vi "Text control 2 v6.1.vi"() -> ()   [LabVIEW 2016]
panel:
  in  "Tab Control":enum32{"Main", "Other parameters"}(tab)
  out "Line running":i32
  out "Total lines":i32
  out "Path":path=path "C:/users/rlp38/09Apr2009LTtesting/test2.txt"
  out "I vs Vg":cluster{"Y data in":dbl[], "X data in":dbl[]}[](graph)
  out "Is max":dbl format="%.2e"
  out "Id max":dbl format="%.2e"
  out "Ig max":dbl format="%.2e"
  out "Imax vs time":cluster{"Y data in":dbl[], "X data in":dbl[]}[](graph)
  out "Imin vs time":cluster{"Y data in":dbl[], "X data in":dbl[]}[](graph)
  out "I vs Vd":cluster{"Y data in":dbl[], "X data in":dbl[]}[](graph)
  in  "Script":string="#pulsedstressV d 0.03 20 0 0.5 0.0827 5\n#\n#itime m\n#gaterangemode a\n#drainrangemode a\n#pulsed on 0.05 0 0.02\n#transfer d -10 40 1 5 40 35\n#transfer d -10 40 1 5 40 35\n#transfer d -10 40 1 5 40 35\n#output d 0 40 20 0 40 1\n#\n#\n#sample 1 0.008 221 6 0.003\n#samplei 400e-6 200 6 0.002 0.1\n#vsu2pulse -10 4\n#\n#stressV 0.016 0.03 2e-4 0.1e-3 11\n#stressI 220e-7 0.08 15\n#transfer s -1 1 0.5 -0.005 0.005 0.005\n#output s 0 0 0 -0.008 0.008 0.002"
  out "Command running:":string
  out "Serial port data":string
  out "Elapsed Time":dbl caption="Elapsed Time (s)"
  in  "Time Units":u16(ring)=1 items=["Seconds", "Minutes", "Hours"]
  in  "Time Offset":dbl caption="Set Start Time (s)"
  in  "Reset":bool
  in  "Auto Reset":bool
  in  "integration time":u32(slide) max=2 step=1 scale=0.0..2.0
  out "Is on":dbl format="%.2e"
  out "Id on":dbl format="%.2e"
  out "Ig on":dbl format="%.2e"
  out "Ion vs time":cluster{"Y data in":dbl[], "X data in":dbl[]}[](graph)
  out "Ioff vs time":cluster{"Y data in":dbl[], "X data in":dbl[]}[](graph)
  out "Ig min":dbl format="%.2e"
  out "Id min":dbl format="%.2e"
  out "Is min":dbl format="%.2e"
  out "Is off":dbl format="%.2e"
  out "Id off":dbl format="%.2e"
  out "Ig off":dbl format="%.2e"
  in  "Integration time (long)":dbl=0.32 min=0.04 max=2.0 step=0.02 format="%.2f"
  in  "Integration time (short)":dbl=0.0019 min=8e-05 max=0.0019 step=8e-05 format="%^.0e"
  in  "Drain: Compliance":dbl=0.001 format="%.8f"
  in  "Gate: Compliance":dbl=0.001 format="%.8f"
  in  "Interrupt run":bool
  in  "Standby":T1
  in  "Full Reset":bool
  in  "SMU4":cluster{"on/off":bool, "Voltage":dbl} {"Voltage" min=-100.0 max=100.0 format="%.2f"}
  in  "Gate Range\nmode":u16(ring) items=["Auto", "Limited", "Fixed"]
  in  "Gate Range":u8(slide)=6 max=11 scale=0.0..11.0
  in  "Source/Drain\nRange mode":u16(ring) items=["Auto", "Limited", "Fixed"]
  in  "Source/Drain Range":u8(slide)=6 max=11 scale=0.0..11.0
  in  "Panel Controls":T2={"Emergency Stop"=refnum, "TransGraph Max"=1e-05, "Text/Graph (text=false)"=TRUE} {"TransGraph Max" format="%.2e"}
  in  "Panel Controls 2":T3={"Emergency Stop"=refnum, "TransGraph Max"=1e-05, "Text/Graph (text=false)"=TRUE, "TransGraph Min"=1e-11} {"TransGraph Min" format="%.2e"; "TransGraph Max" format="%.2e"}
  out "error out":errorcluster
  in  "Delay before read (ms)":u32=1000
  in  "byte count":u32=64
  in  "Serial End Mode for Reads":u16(ring)=2 items=["None", "LastBit", "TermChar"]
  in  "Timeout (ms)":u32=10000
  in  "Enable Termination\nChar (T)":bool=TRUE
  in  "Termination char\n(0xA = '\\n' = LF)\n(0xD = '\\r' = CR)":u8=13 format="%.0x"
  in  "flow control":u16(ring) items=["None"=0, "XON/XOFF"=1, "RTS/CTS"=2, "DTR/DSR"=4]
  in  "stop bits":u16(ring)=10 items=["1.0"=10, "1.5"=15, "2.0"=20]
  in  "parity":u16(ring) items=["None", "Odd", "Even", "Mark", "Space"]
  in  "data bits":u16=8 min=5 max=8 step=1
  in  "VISA resource name":refnum<visa-resource-name>="COM6"
  in  "baud rate":u32=9600
  out "Timings Indicator":T4
  in  "Timings (overwritten by the Front Panel)":T5={"integration time"=0, "Short/Long integration time"=0.00064, "hold time (sec)"=0.0, "delay time (sec)"=0.0, "Step Time (0 disables)"=0.0, "sweep method"=0, "Pulse period"=0.005, "Base voltage"=0.0, "Pulse width"=0.0005} {"Pulse width" min=0.0005 max=0.1 step=0.0001 format="%.4f"; "Base voltage" format="%^.4e"; "Pulse period" min=0.005 max=1.0 step=0.0001 format="%.4f"; "sweep method" items=["Continuous", "Pulsed"]; "Step Time (0 disables)" format="%.2f"; "delay time (sec)" format="%.4f"; "hold time (sec)" format="%.4f"; "Short/Long integration time" format="%^.0e"; "integration time" scale=0.0..2.0}
  in  "Gate":T6={"Gate Start"=0.0, "Gate Stop"=2.0, "Gate Step (linear only)"=1.0, "Gate Compliance"=0.0001, "Gate PComp"=0.0, "Range mode"=0, "Range"=6} {"Range" max=11 scale=0.0..11.0; "Range mode" items=["Auto", "Limited", "Fixed"]; "Gate PComp" format="%^.2e"; "Gate Compliance" format="%^.2e"; "Gate Step (linear only)" format="%^.4e"; "Gate Stop" format="%^.4e"; "Gate Start" format="%^.4e"}
  in  "Drain 2":T7={"Drain Start"=0.0, "Drain Stop"=2.0, "Drain Compliance"=0.0001, "Drain Step"=1.0, "Drain PComp"=0.0, "Range mode"=0, "Range"=6} {"Range" max=11 scale=0.0..11.0; "Range mode" items=["Auto", "Limited", "Fixed"]; "Drain PComp" format="%^.2e"; "Drain Step" format="%^.4e"; "Drain Compliance" format="%^.2e"; "Drain Stop" format="%^.4e"; "Drain Start" format="%^.4e"}
  # "Time"
  # "Syntax:\nitime [s|m|l] time(sec): [s|m|l] determines the integration time setting (small|medium|long) and time sets the value.\nNOTE: The value of the integration time has to be within the range allowed by its category (s|m|l), otherwise, the closest value will be used. (e.g. if the category is set to short but the time value is very long, the actual value used will be the maximum short integration time.\nIntegration times:\n    Short: Default: 640 us. Range: 8E-5 - 1.92E-3 seconds.\n    Medium: Fixed at 1 NPL cycle (0.02 seconds).\n    Long: Default: 16 NPL cycles (0.32 seconds). Range: 2-100 NPL cycles (0.04 seconds - 2 seconds).\ngaterangemode [a|l|f]\ndrainrangemode [a|l|f]\npulsed [on|off] PulsePeriod(sec) PulseBaseVoltage PulseONWidth(sec)\nstandby [on l off]\nwait NumMilliseconds\nwait-min NumMinutes\n# texthere = comment\ntransfer [s|d] VgStart VgStop VgStep VdStart VdStop VdStep\noutput [s|d] VgStart VgStop VgStep VdStart VdStop VdStep\nsample Vg Vd NumSamples Time(s) SampleInterval(s)\nsamplei Idg NumSamples Time(s) SampleInterval(s) VDGcompliance\n100 samples is approximately 13 seconds with medium integration\n# if in doubt use SampleInterval(s) = 0.004\nstressV VG VD IGcompliance IDcompliance Duration(sec)\nstressI IDG VDGcompliance Duration(sec)\nvsu2pulse Bias Duration(s)\npulsedstressV [s|d] VEstop VgON VgOFF Period(s) PulseONwidth(s) Vd\nsample-fpp Vg Vd NumSamples Time\nresample-fpp Vg Vd\ntransfer-fpp [s|d] VgStart VgStop VgStep VdStart VdStop VdStep\noutput-fpp [s|d] VgStart VgStop VgStep VdStart VdStop VdStep\nserial SerialPortCommand"
  # "1\n2\n3\n4\n5\n6\n7\n8\n9\n10\n11\n12\n13\n14\n15\n16\n17\n18\n19\n20"
  # "Serial port settings"
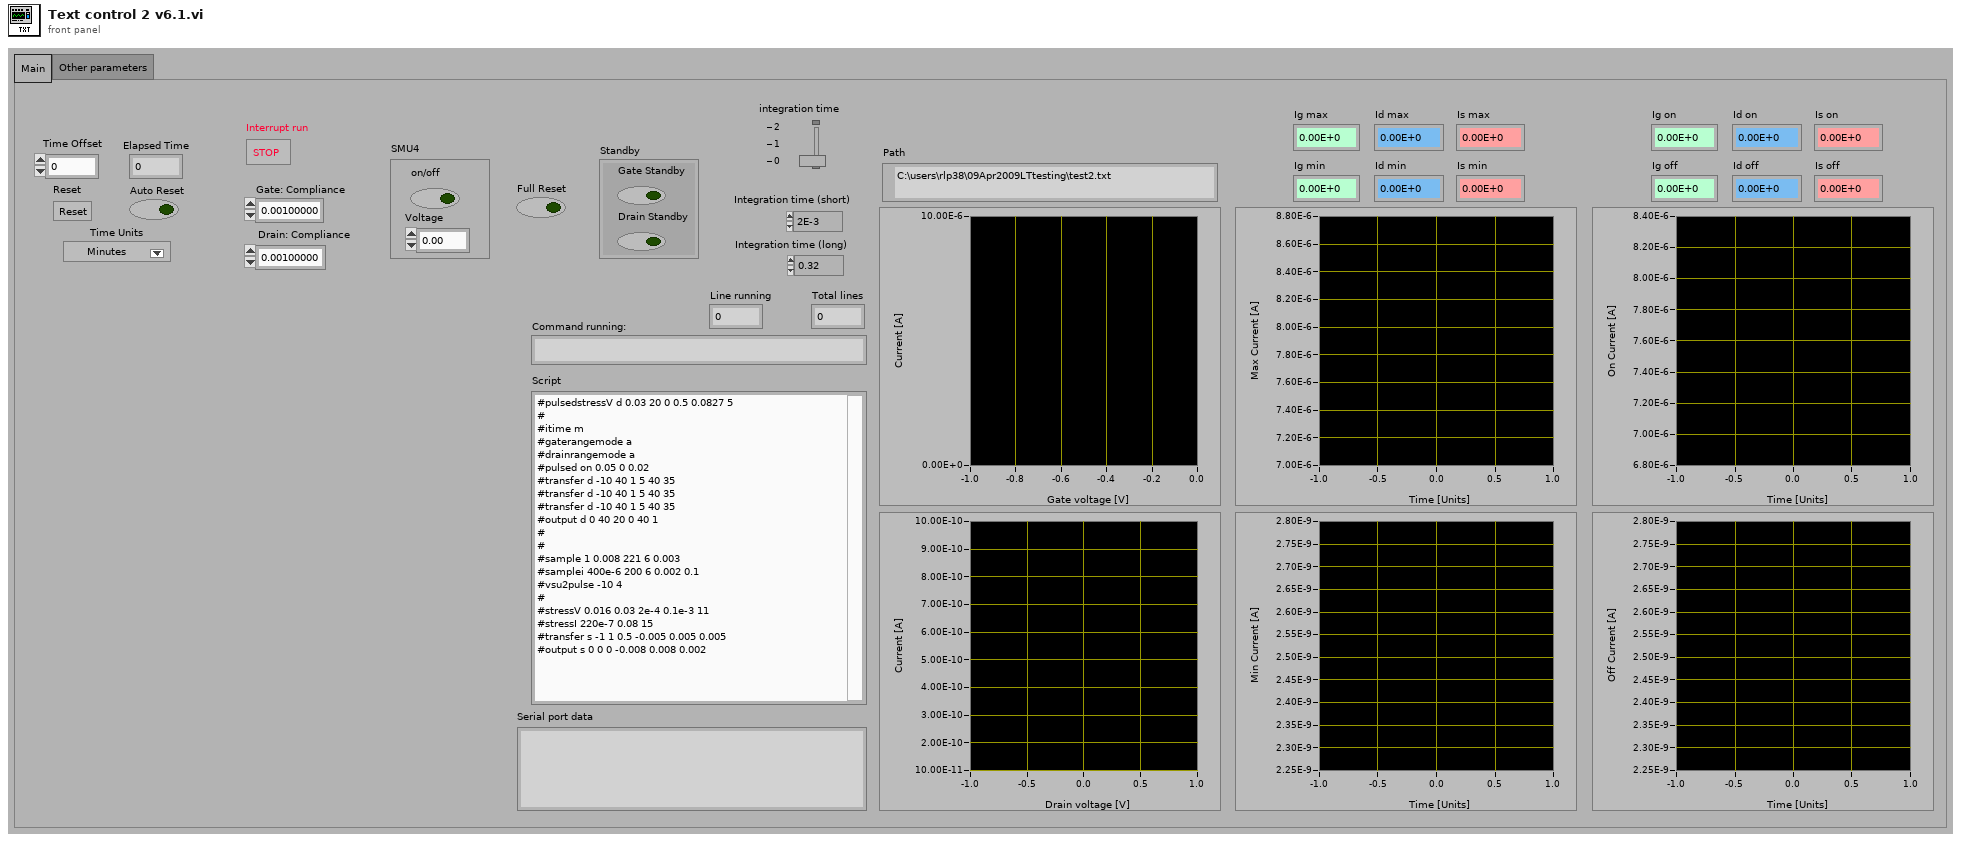
[diagram p1: front panel]
types:
  T1 = cluster{"Gate Standby":bool, "Drain Standby":bool}
  T2 = cluster{"Emergency Stop":refnum<vi>, "TransGraph Max":dbl, "Text/Graph (text=false)":bool}
  T3 = cluster{"Emergency Stop":refnum<vi>, "TransGraph Max":dbl, "Text/Graph (text=false)":bool, "TransGraph Min":dbl}
  T4 = cluster{"integration time (0:s, 1:m, 2:l)":u32, "Short/Long integration time":dbl, "hold time (sec)":dbl, "delay time (sec)":dbl, "Step Time (0 disables)":dbl, "sweep method":u16, "Pulse period":dbl, "Base voltage":dbl, "Pulse width":dbl}
  T5 = cluster{"integration time":u32, "Short/Long integration time":dbl, "hold time (sec)":dbl, "delay time (sec)":dbl, "Step Time (0 disables)":dbl, "sweep method":u16, "Pulse period":dbl, "Base voltage":dbl, "Pulse width":dbl}
  T6 = cluster{"Gate Start":dbl, "Gate Stop":dbl, "Gate Step (linear only)":dbl, "Gate Compliance":dbl, "Gate PComp":dbl, "Range mode":u16, "Range":u8}
  T7 = cluster{"Drain Start":dbl, "Drain Stop":dbl, "Drain Compliance":dbl, "Drain Step":dbl, "Drain PComp":dbl, "Range mode":u16, "Range":u8}
  T8 = enum16{"open", "replace", "create", "open or create", "replace or create", "replace or create with confirmation"}
  T9 = cluster{"V2 Start":dbl, "V2 Step":dbl, "Number of points":i32}
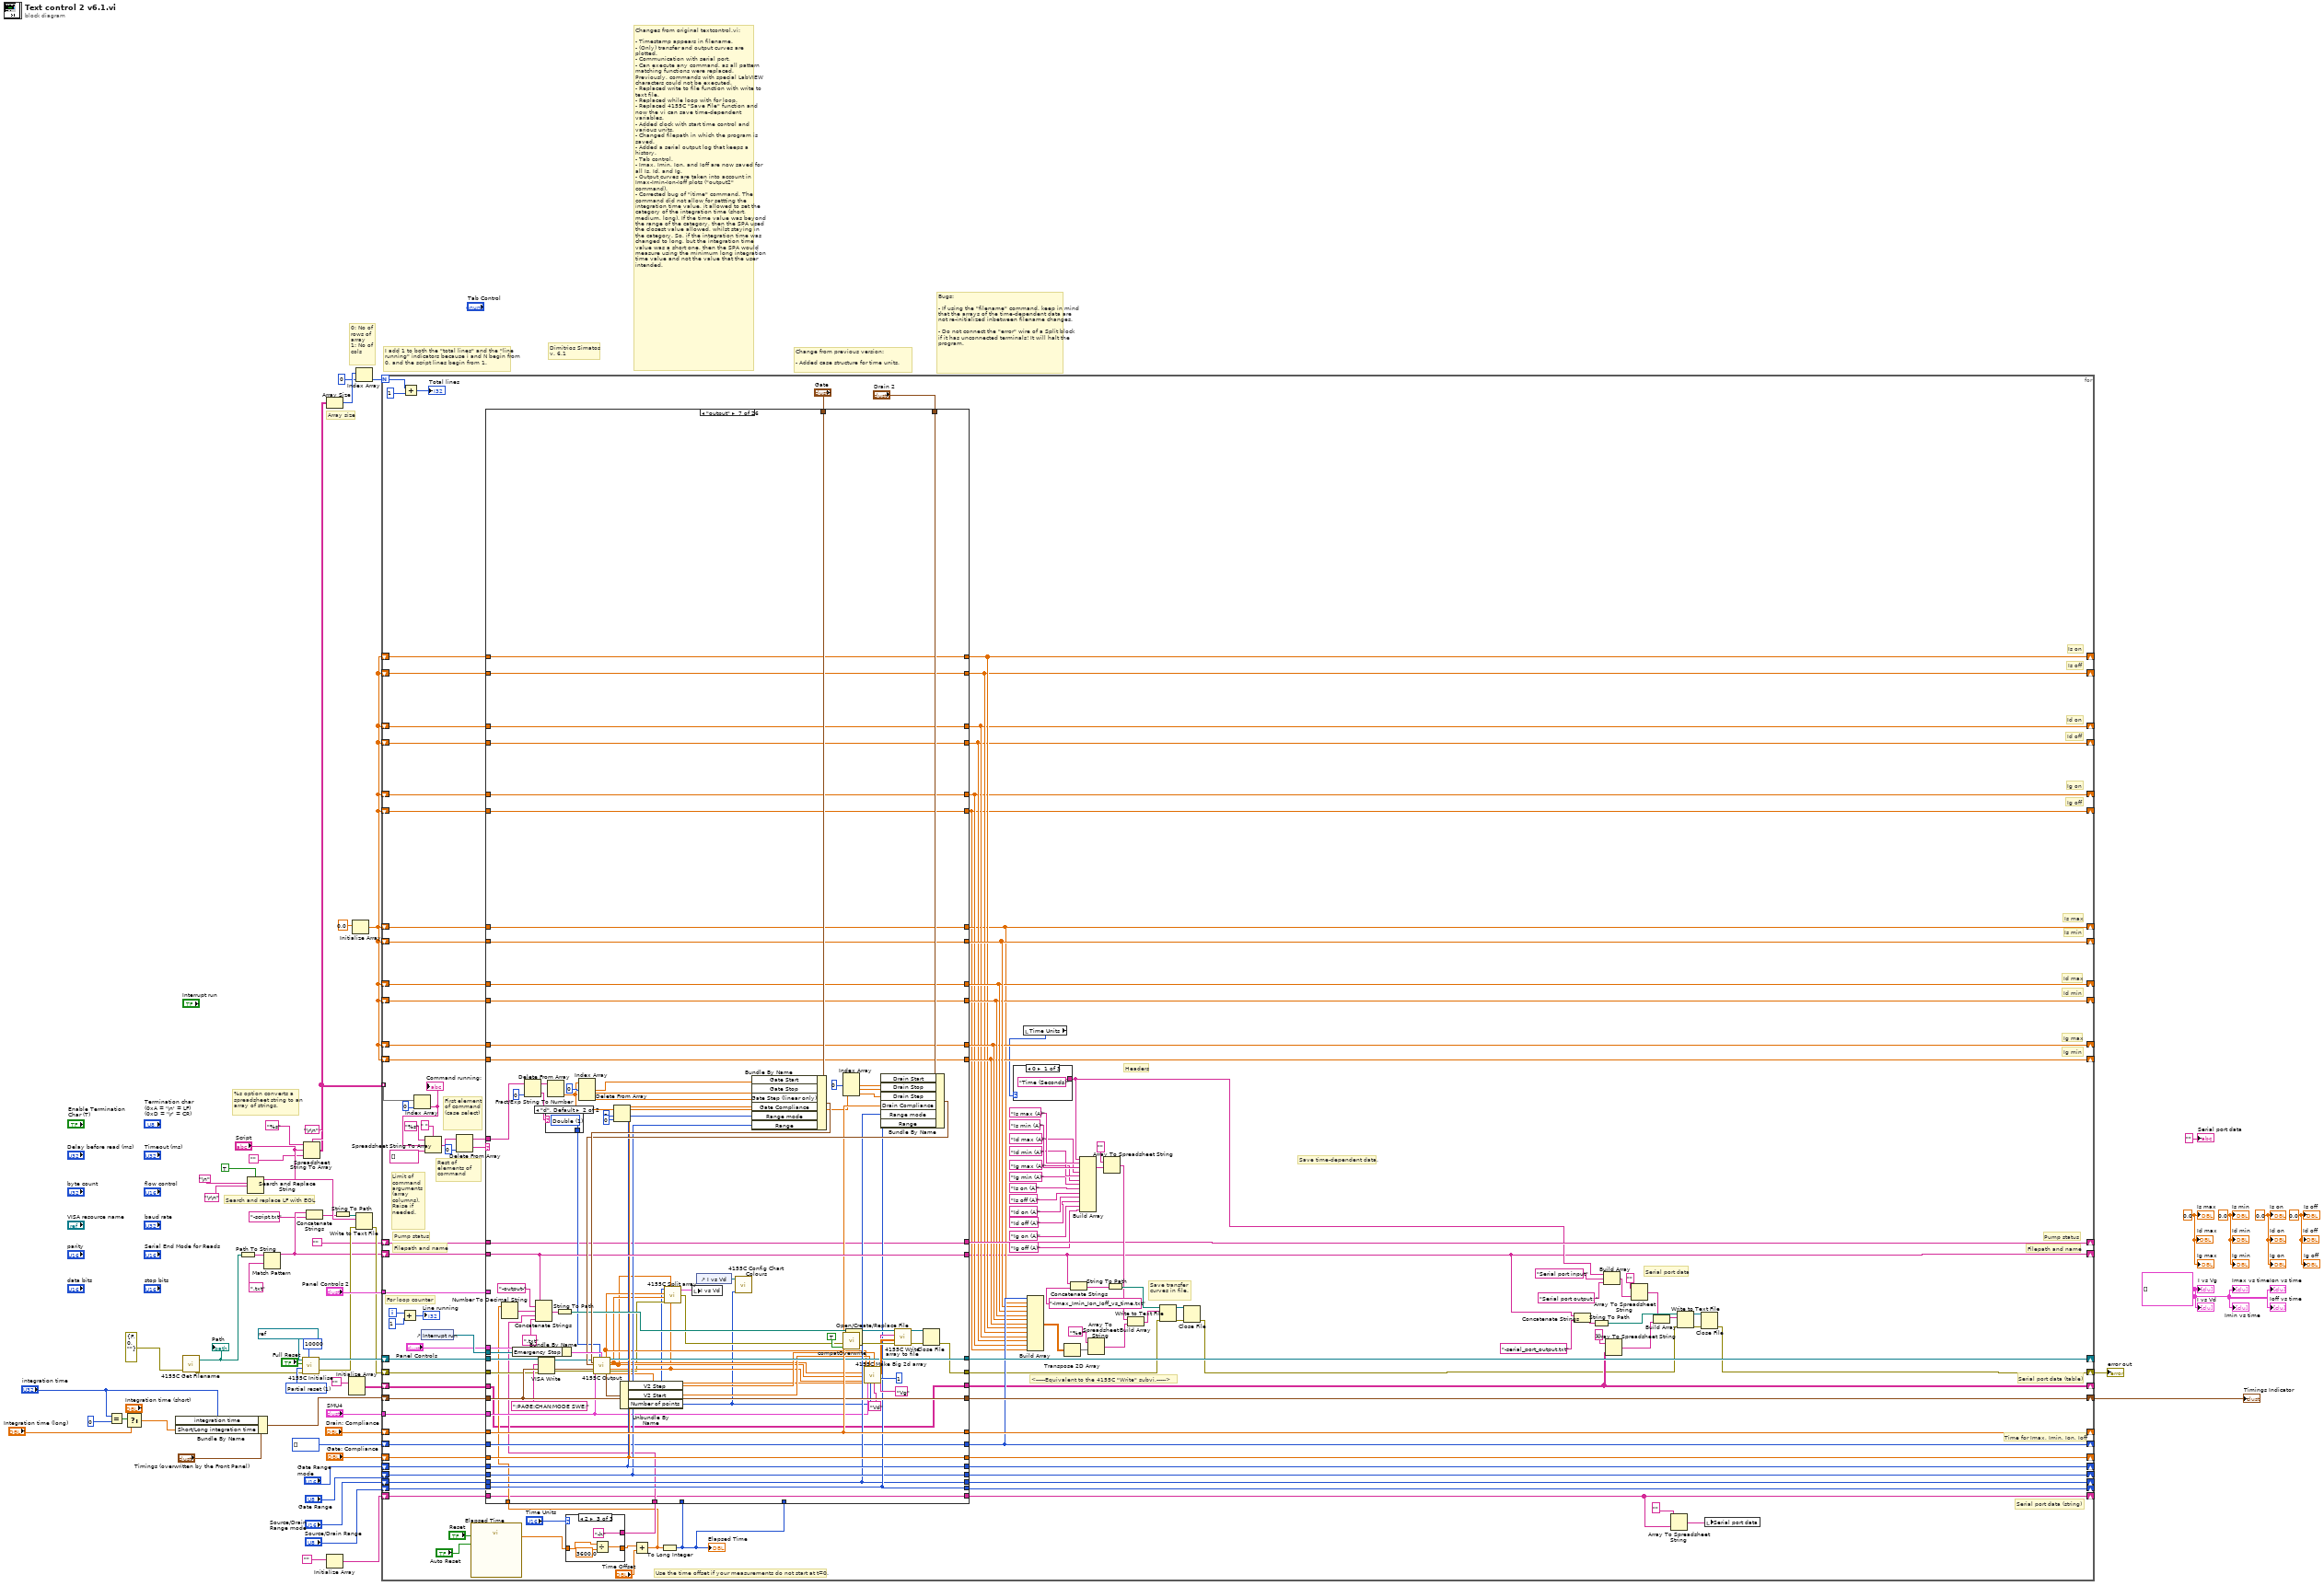
[diagram p0: block diagram]
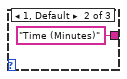
[diagram p2: hidden frame]
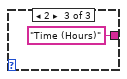
[diagram p3: hidden frame]
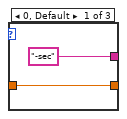
[diagram p4: hidden frame]
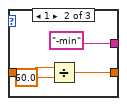
[diagram p5: hidden frame]
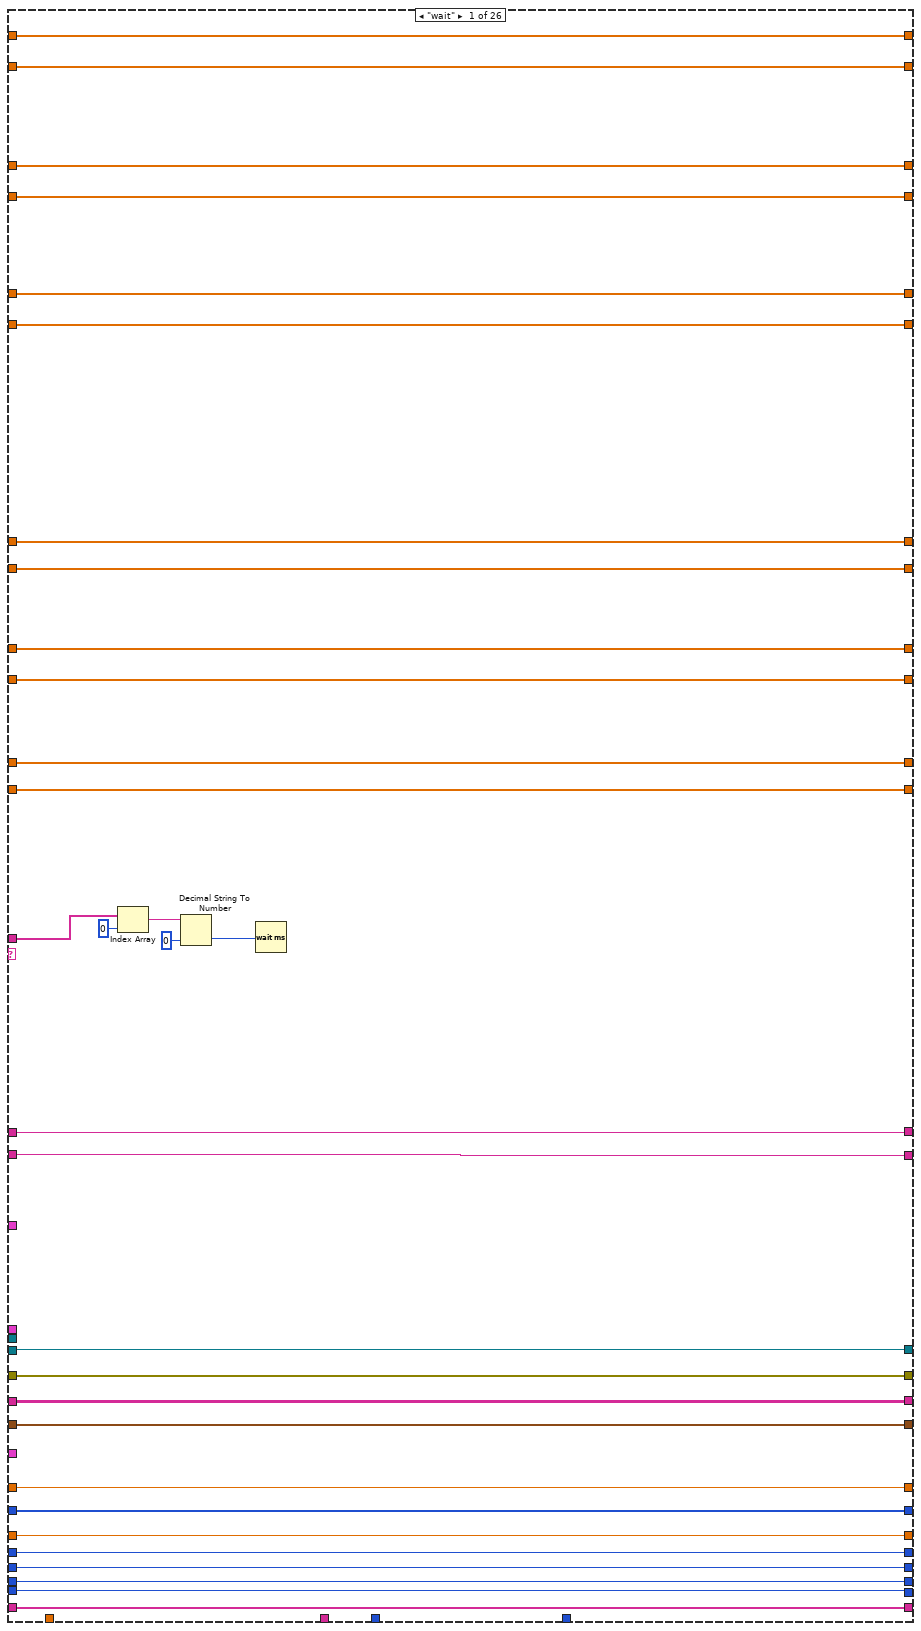
[diagram p6: hidden frame]
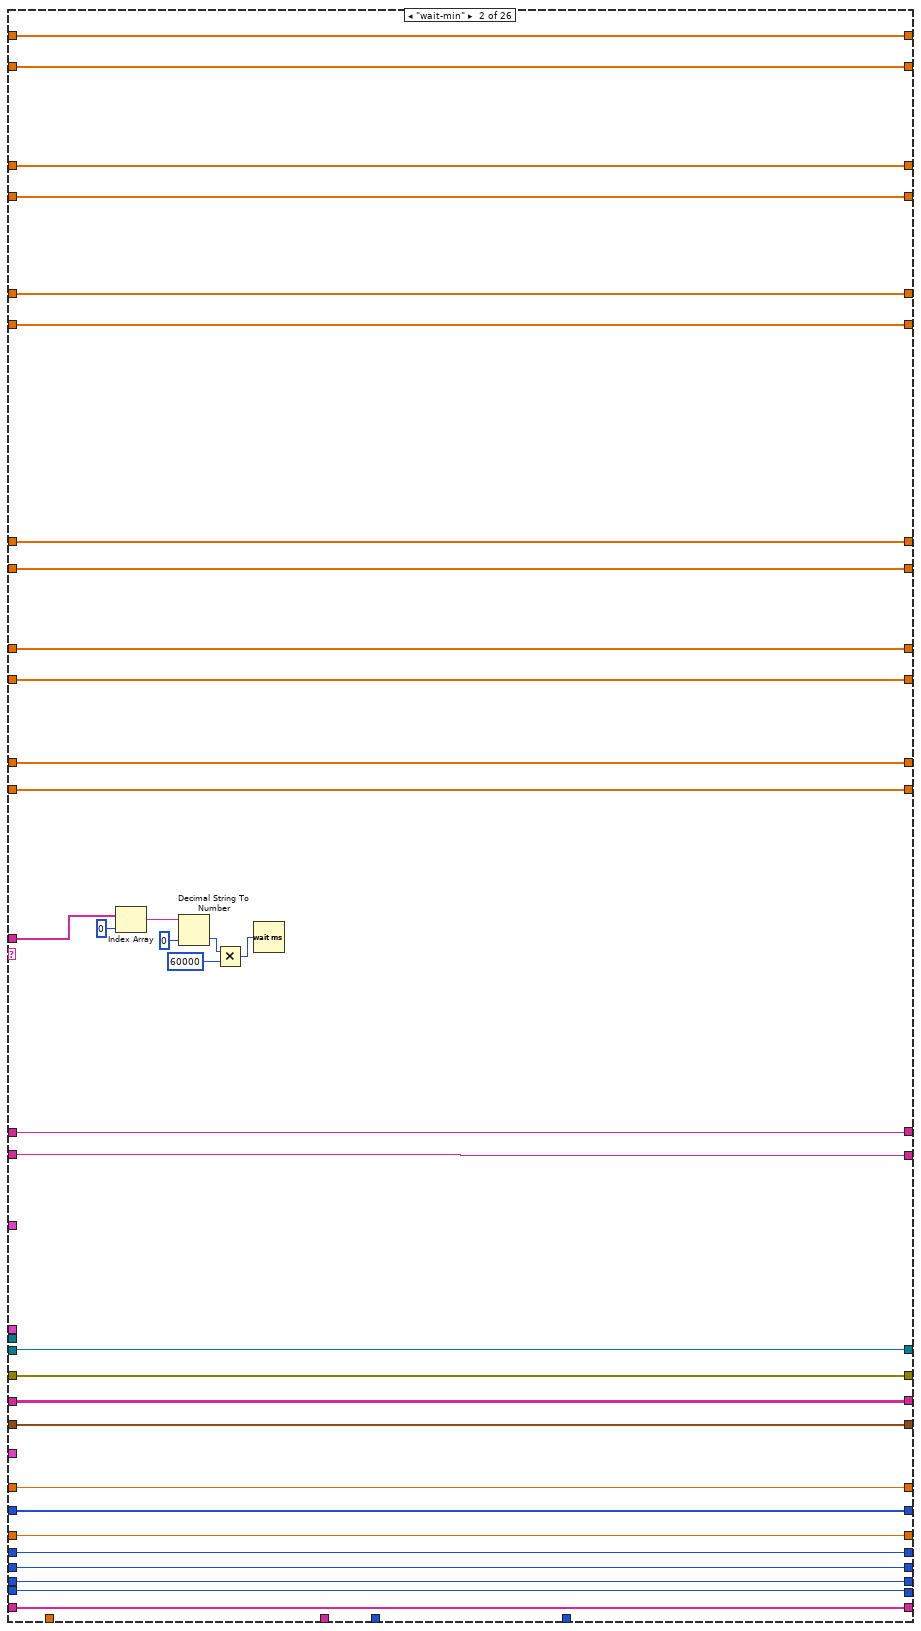
[diagram p7: hidden frame]
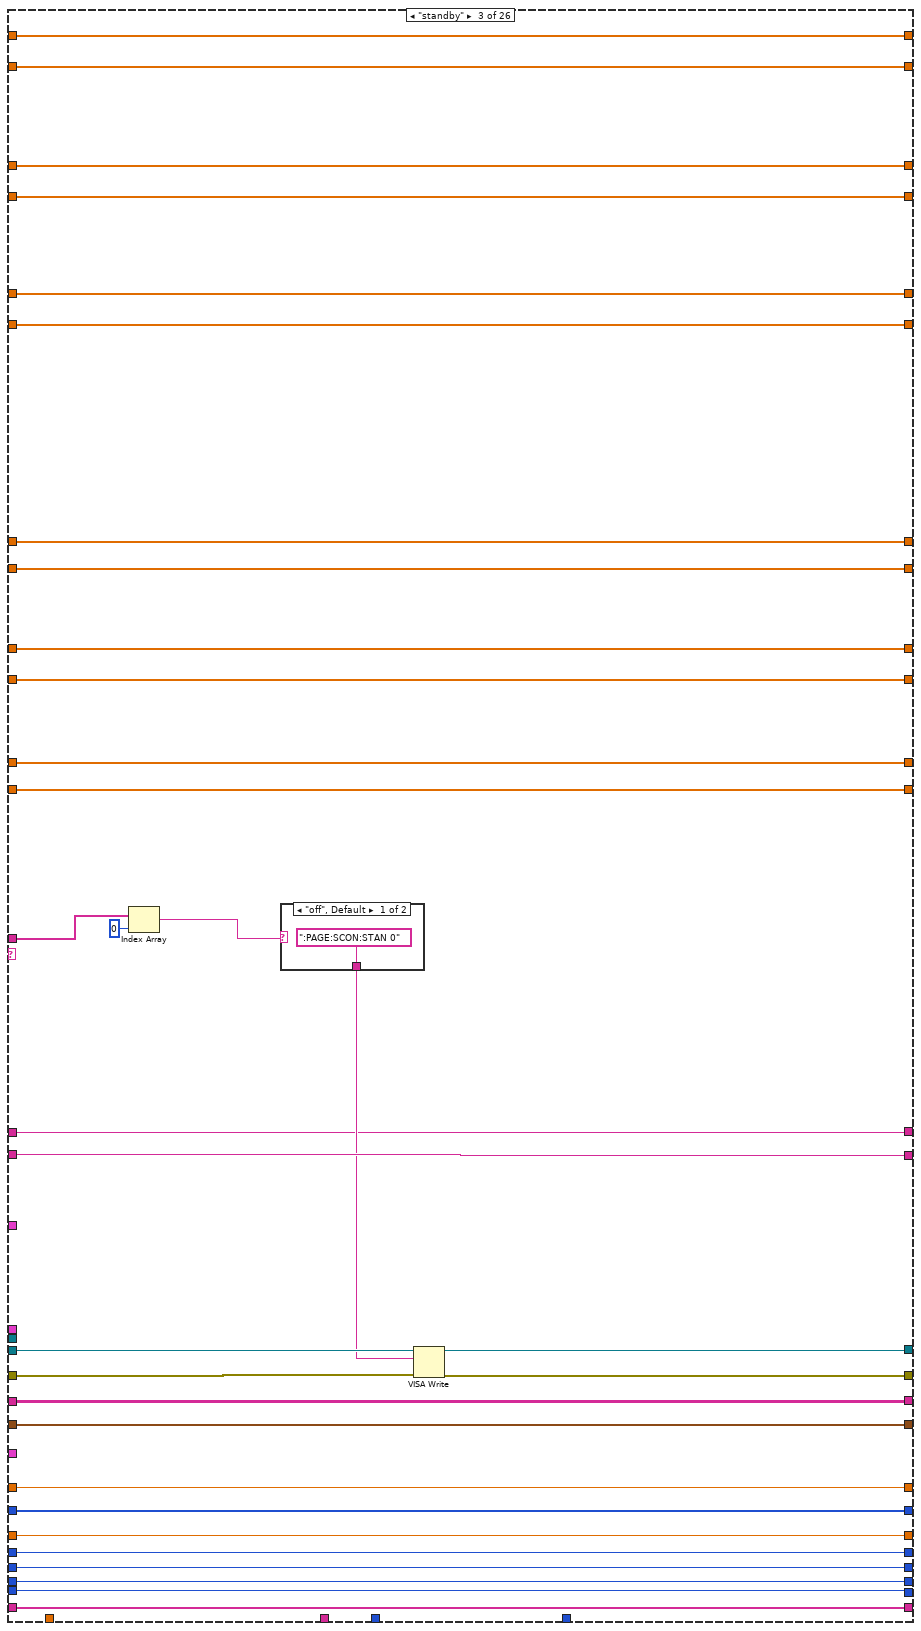
[diagram p8: hidden frame]
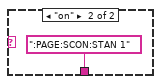
[diagram p9: hidden frame]
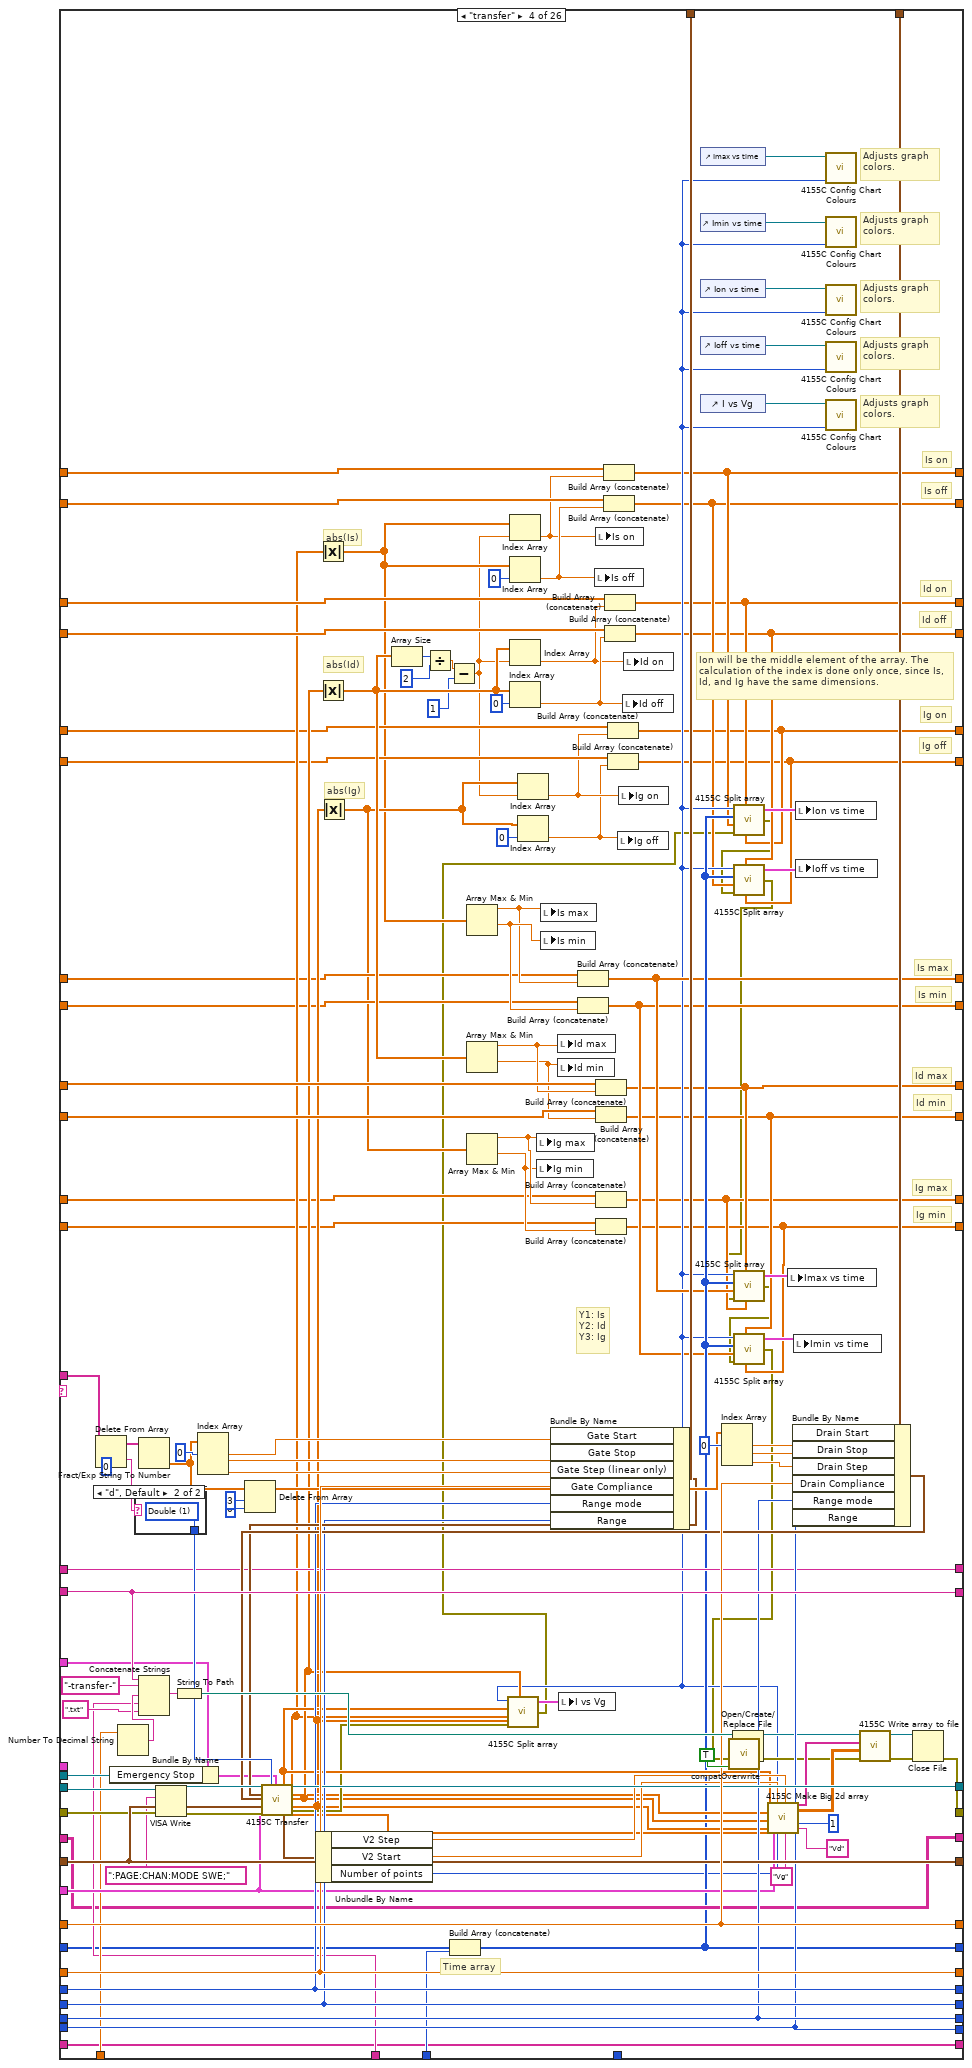
[diagram p10: hidden frame]
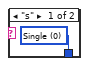
[diagram p11: hidden frame]
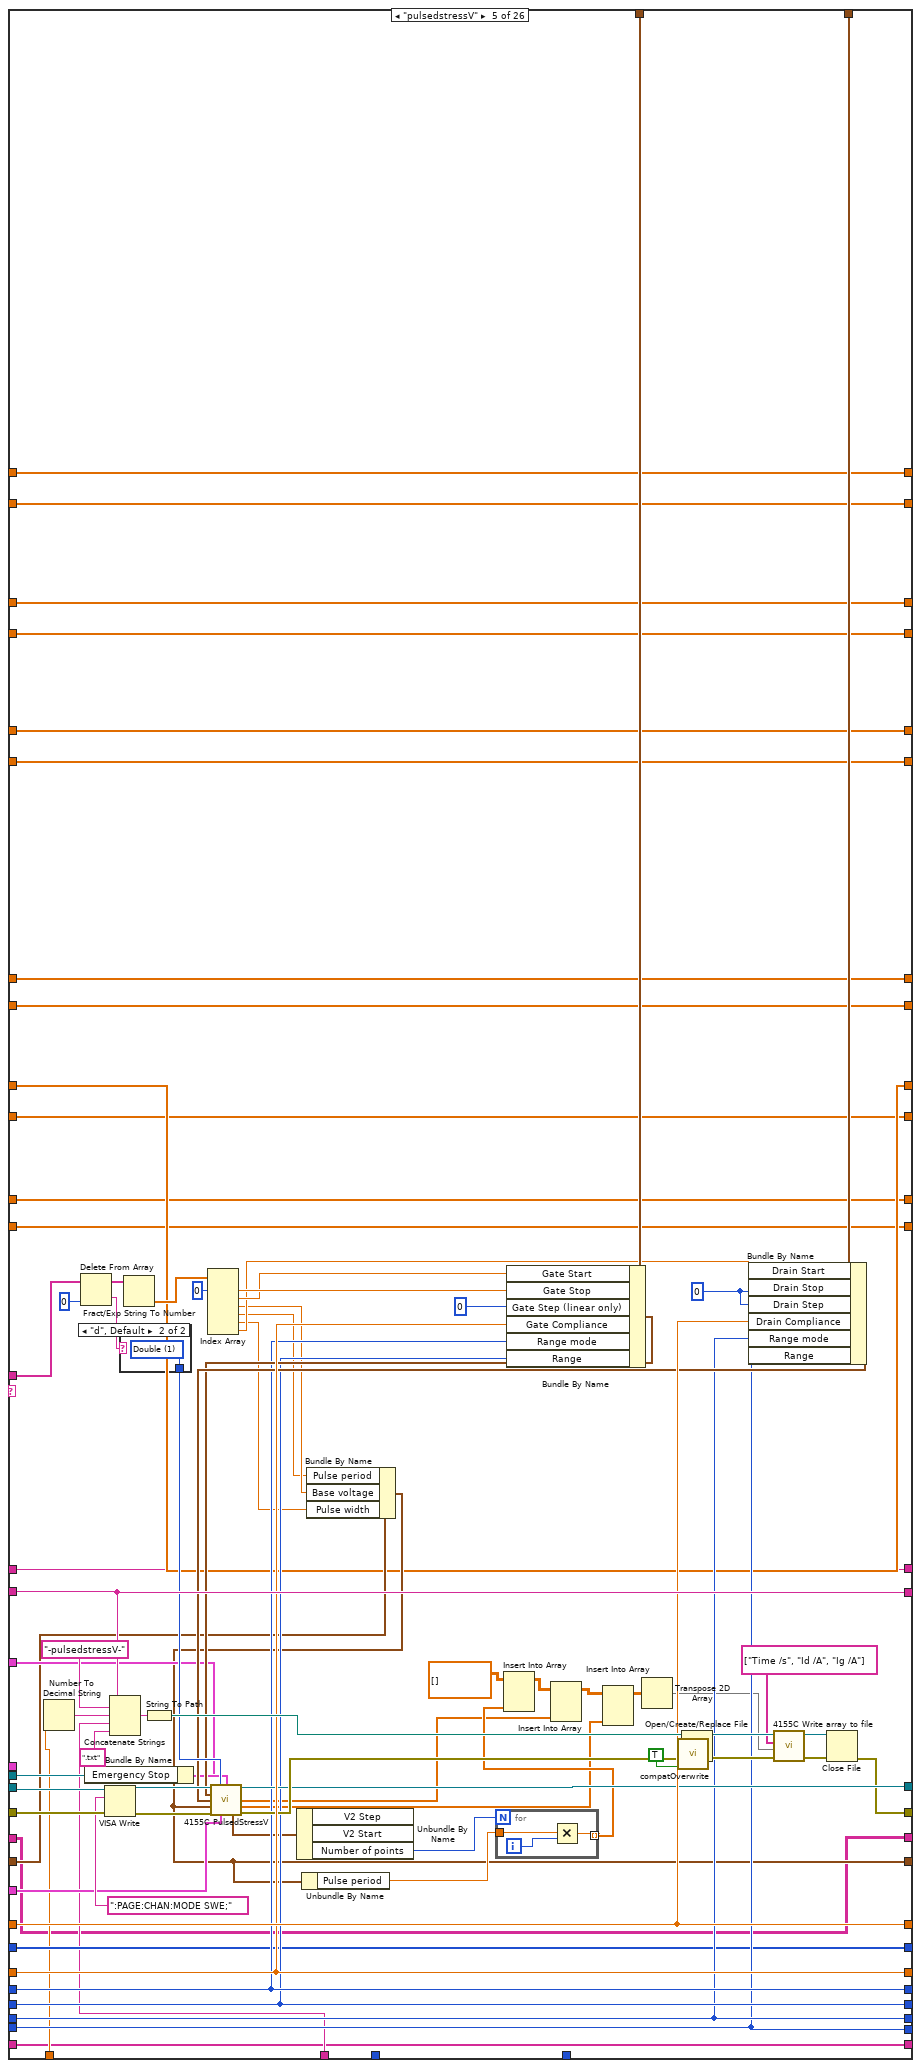
[diagram p12: hidden frame]
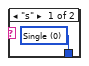
[diagram p13: hidden frame]
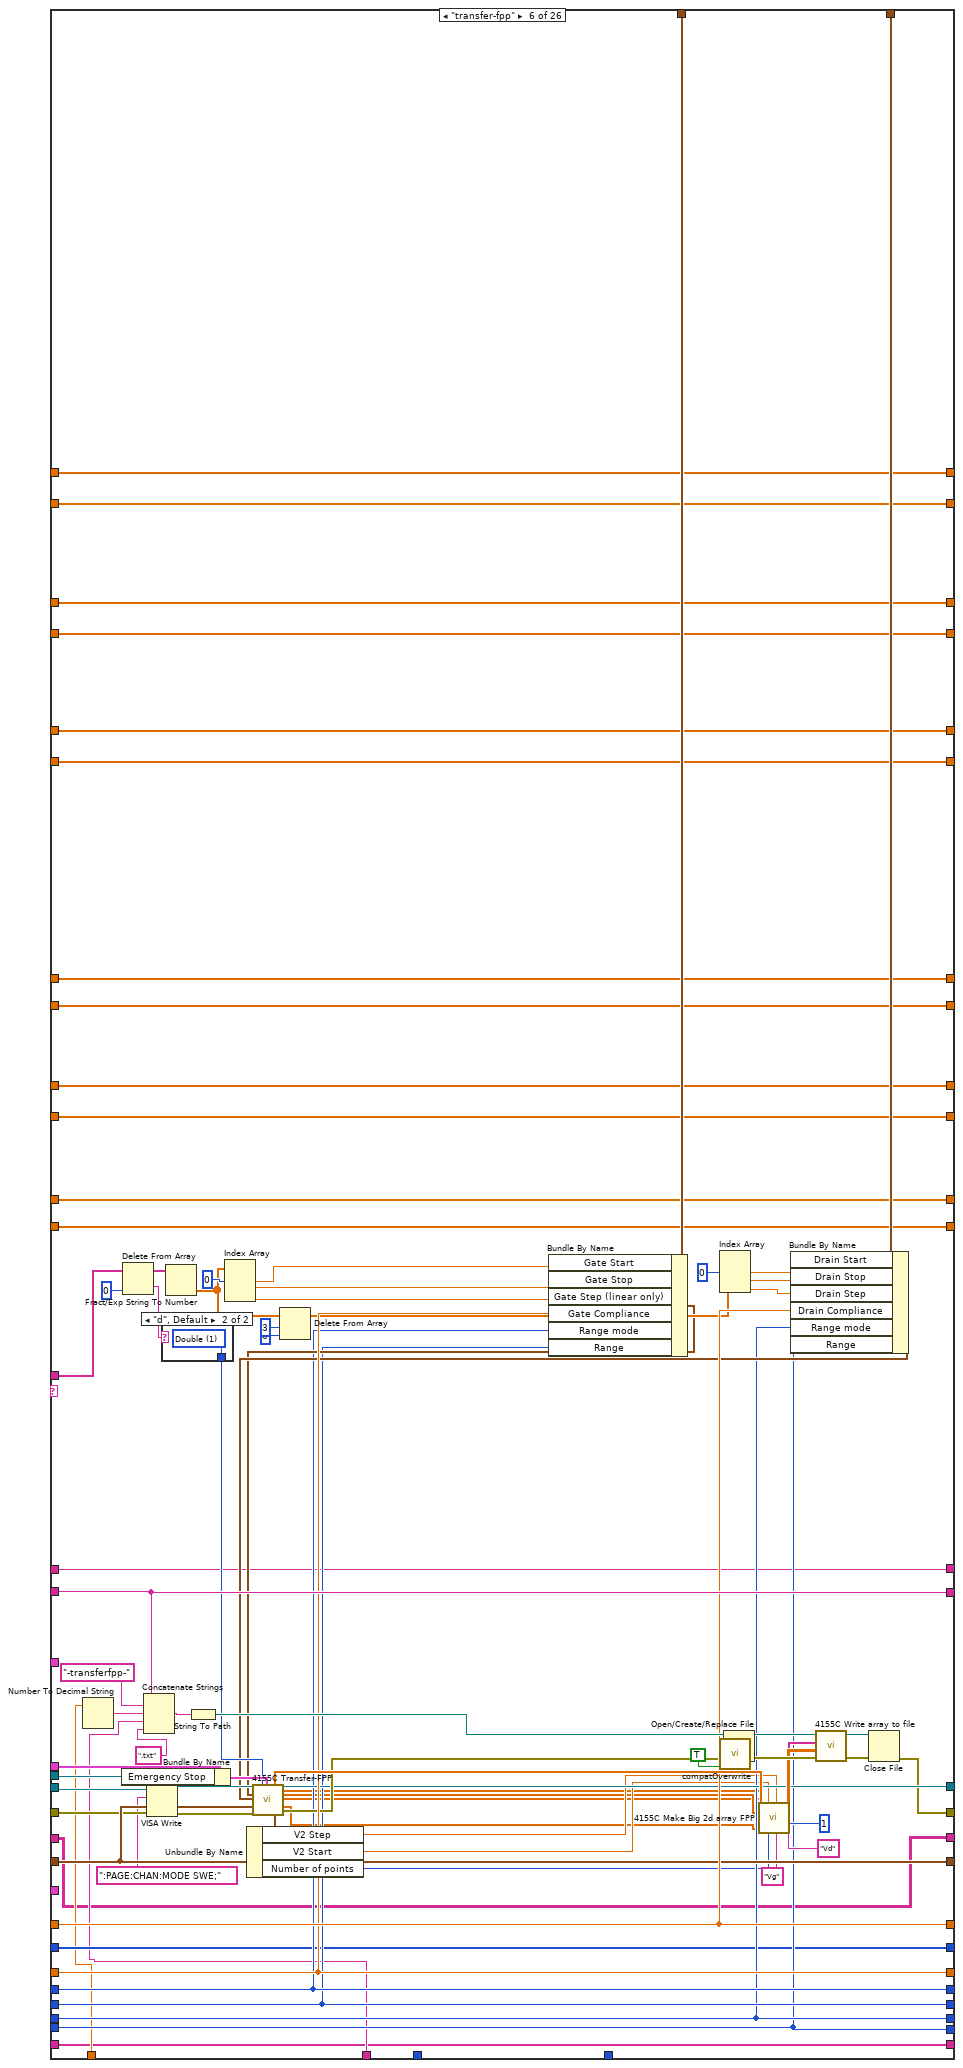
[diagram p14: hidden frame]
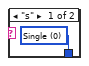
[diagram p15: hidden frame]
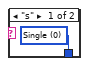
[diagram p16: hidden frame]
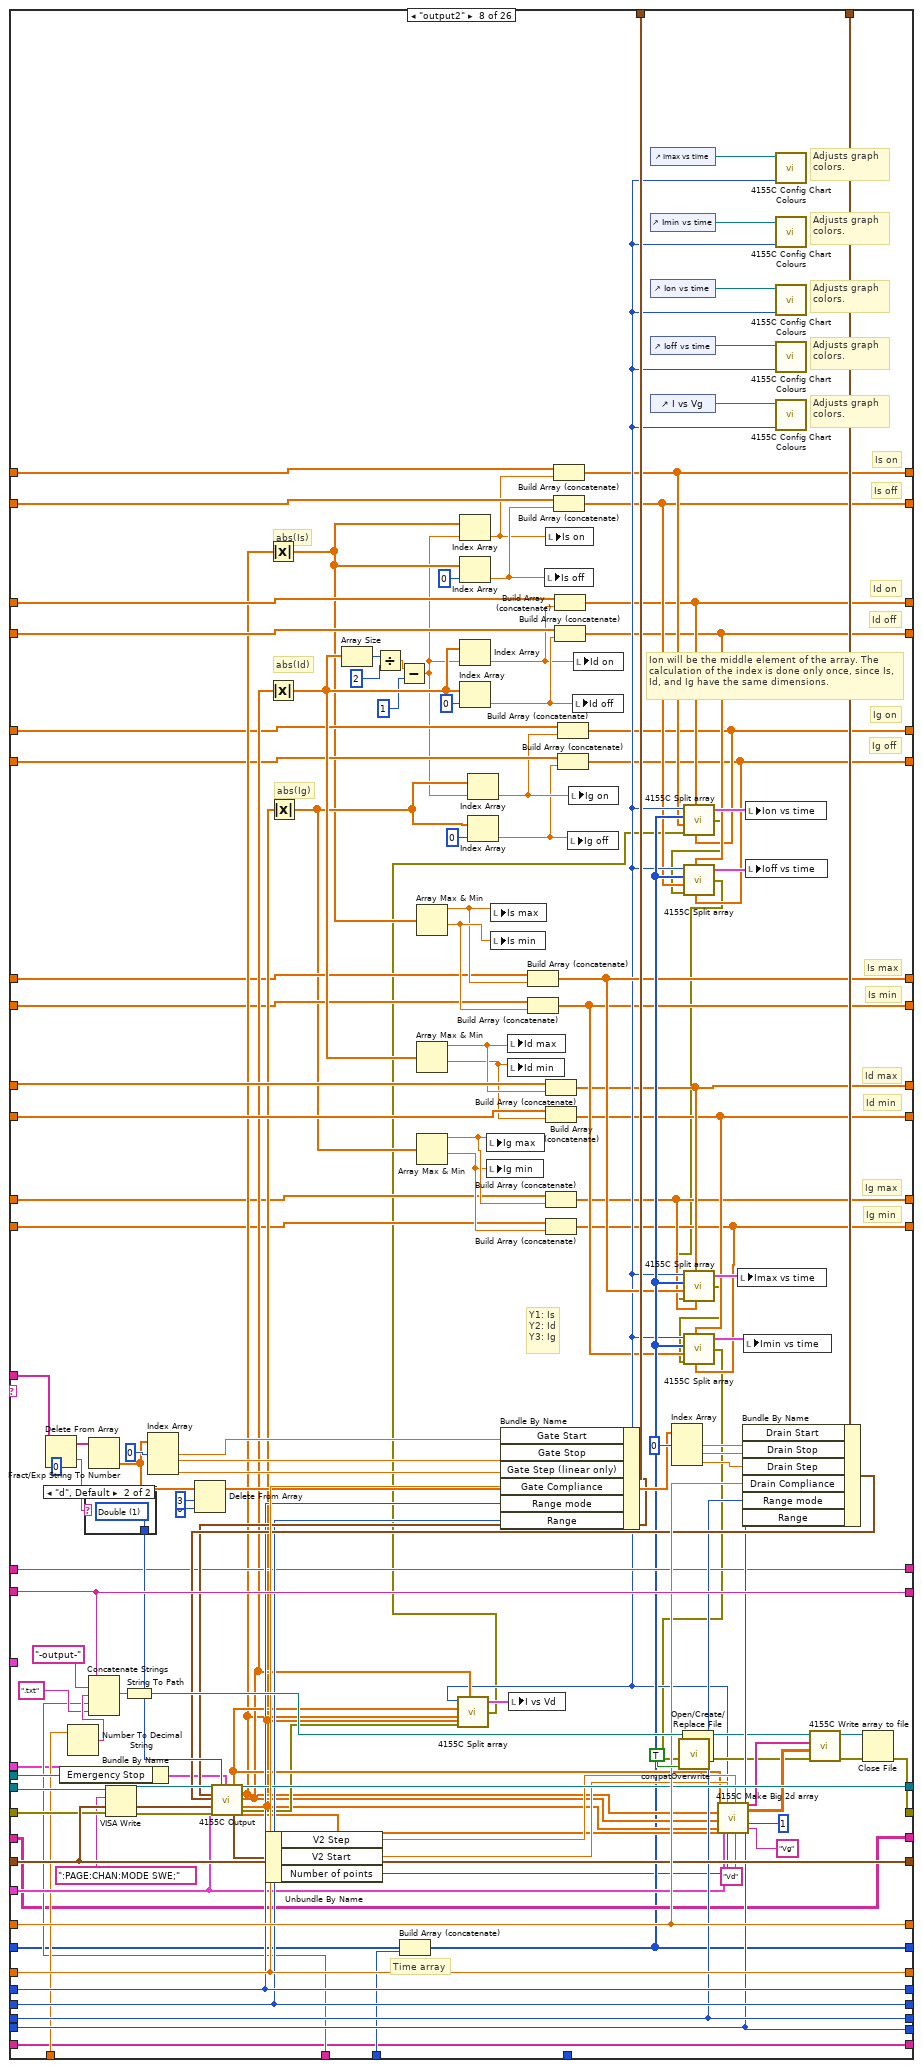
[diagram p17: hidden frame]
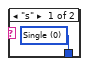
[diagram p18: hidden frame]
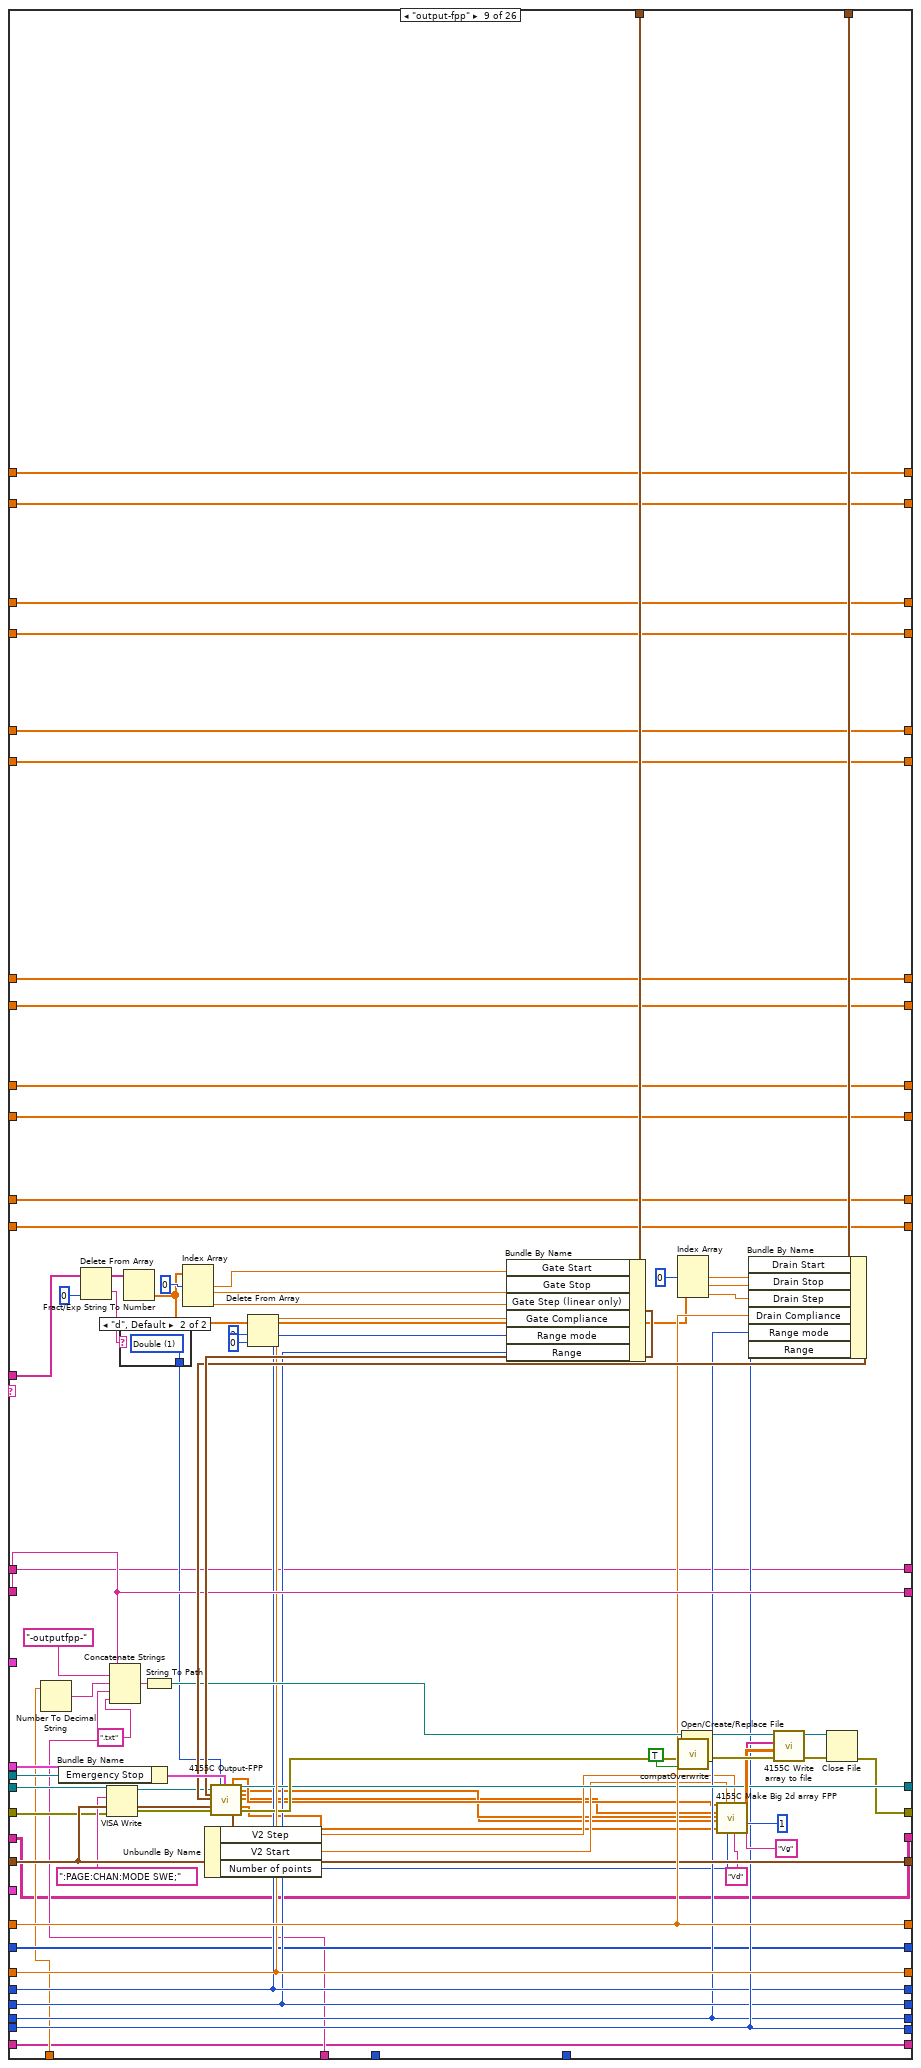
[diagram p19: hidden frame]
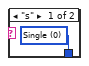
[diagram p20: hidden frame]
diagram:
  w2 = cluster{"Y data in":dbl[], "X data in":dbl[]}[] [] ("I vs Vg")
  w3 = 0.0 ("Is off")
  w4 = 0.0 ("Is on")
  w5 = 0.0 ("Is min")
  w6 = 0.0 ("Is max")
  w55 = u16 1 items=["Reset All", "Partial reset"] ("Type of reset")
  # "Change from previous version:\n\n- Added case structure for time units."
  # "I add 1 to both the \"total lines\" and the \"line running\" indicators because i and N begin from 0, and the script lines begin from 1."
  # "Bugs:\n\n- If using the \"filename\" command, keep in mind that the arrays of the time-dependent data are not re-initialized inbetween filename changes. \n\n- Do not connect the \"error\" wire of a Split block if it has unconnected terminals! It will halt the program."
  # "Array size"
  # "%s option converts a spreadsheet string to an array of strings."
  # "0: No of rows of array\n1: No of cols"
  # "Dimitrios Simatos\nv. 6.1"
  # "Changes from original textcontrol.vi:\n\n- Timestamp appears in filename.\n- (Only) transfer and output curves are plotted.\n- Communication with serial port.\n- Can execute any command, as all pattern matching functions were replaced. Previously, commands with special LabVIEW characters could not be executed.\n- Replaced write to file function with write to text file.\n- Replaced while loop with for loop.\n- Replaced 4155C \"Save File\" function and now the vi can save time-dependent variables.\n- Added clock with start time control and various units.\n- Changed filepath in which the program is saved.\n- Added a serial output log that keeps a history.\n- Tab control.\n- Imax, Imin, Ion, and Ioff are now saved for all Is, Id, and Ig.\n- Output curves are taken into account in Imax-Imin-Ion-Ioff plots (\"output2\" command).\n- Corrected bug of \"itime\" command. The command did not allow for settting the integration time value, it allowed to set the category of the integration time (short, medium, long). If the time value was beyond the range of the category, then the SPA used the closest value allowed, whilst staying in the category. So, if the integration time was changed to long, but the integration time value was a short one, then the SPA would measure using the minimum long integration time value and not the value that the user intended."
  # "Search and replace LF with EOL"
  n1 = Equal?(x="integration time", y=u32 0) -> (x = y?=w56:bool)
  n2 = Select(t="Integration time (short)", s=w56, f="Integration time (long)") -> (s? t:f=w11:dbl)
  n3 = Bundle By Name(cluster="Timings (overwritten by the Front Panel)", "integration time"="integration time", "Short/Long integration time"=w11) -> (w48:T5)
  n4 = call "4155C Get Filename.vi"("error in (no error)"=errorcluster {"status"=FALSE, "code"=0, "source"=""}) -> ("error out"=w50:errorcluster, "path"=w25:path)  [unwired: 2 in, 1 out]
  "Path" <- w25
  n5 = Path To String(path=w25) -> (string=w26:string)
  n6 = Search and Replace String(replace all?=TRUE ("replace all? (F)"), input string="Script", search string="\n", replace string="\r\n") -> (result string=w38:string)  [unwired: 4 in, 3 out]
  n7 = Match Pattern(string=w26, regular expression=".txt") -> (before substring=w9:string)  [unwired: 1 in, 3 out]
  n8 = call "4155C Initialise.vi"("VISA resource name in"=refnum<visa-resource-name> "GPIB0::14::INSTR", "Reset"="Full Reset", "Type of reset"=w55, "error in (no error)"=w50, "VISA Timeout Value"=u32 10000) -> ("VISA Resource Name out"=w49:refnum<visa-resource-name>, "error out"=w21:errorcluster)
  n9 = Spreadsheet String To Array(delimiter (Tab)="\r\n", format string="%s", spreadsheet string="Script", array type (2D Dbl)="") -> (array=w29:string[][])
  n10 = Concatenate Strings(w9, "-script.txt" ("string")) -> (w10:string)
  n11 = Array Size(array=w29) -> (size(s)=w33:i32[])
  n12 = Initialize Array("") -> (w16:string[])  [unwired: 1 in]
  n13 = String To Path(string=w10) -> (path=w22:path)
  n14 = Initialize Array("") -> (w14:string[][])  [unwired: 2 in]
  n15 = Initialize Array(0.0 ("element")) -> (w18:dbl[])  [unwired: 1 in]
  n16 = Index Array(array=w33, index=0) -> (element=w31:i32)
  n17 = Write to Text File(file (use dialog)=w22, text=w38, error in=w21) -> (error out=w20:errorcluster)  [unwired: 1 in, 2 out]
  n18 = for {
    N: w31 -> [w129]
    tunnel: "SMU4" -> [w165]
    shift-left: "Source/Drain Range" -> [w170]
    shift-right: [w166] -> _
    shift-left: "Source/Drain\nRange mode" -> [w171]
    shift-right: [w167] -> _
    shift-left: "Gate Range" -> [w172]
    shift-right: [w168] -> _
    shift-left: "Gate Range\nmode" -> [w173]
    shift-right: [w169] -> _
    shift-left: "Gate: Compliance" -> [w182]
    shift-right: [w178] -> _
    shift-left: "Drain: Compliance" -> [w183]
    shift-right: [w179] -> _
    shift-left: w48 -> [w184]
    shift-right: [w180] -> w12
    shift-left: w20 -> [w185]
    shift-right: [w63] -> w24
    shift-left: w49 -> [w186]
    shift-right: [w181] -> _
    shift-left: w9 -> [w187]
    shift-right: [w66] -> _
    tunnel: "Panel Controls 2" -> [w164]
    shift-right: [w78] -> _
    shift-left: w18 -> [w163]
    shift-right: [w114] -> _
    shift-left: i32[] [] -> [w159]
    tunnel: w29 -> [w158] mode=indexing
    shift-right: [w77] -> _
    shift-left: w18 -> [w135]
    shift-right: [w108] -> _
    shift-left: w16 -> [w121]
    shift-right: [w116] -> _
    shift-left: "" -> [w115]
    shift-right: [w109] -> _
    shift-left: w14 -> [w111]
    shift-right: [w71] -> _
    shift-left: w18 -> [w99]
    shift-right: [w72] -> _
    shift-left: w18 -> [w98]
    shift-right: [w76] -> _
    shift-left: w18 -> [w87]
    shift-right: [w75] -> _
    shift-left: w18 -> [w86]
    shift-right: [w69] -> _
    shift-left: w18 -> [w85]
    shift-right: [w79] -> _
    shift-left: w18 -> [w84]
    shift-right: [w70] -> _
    shift-left: w18 -> [w83]
    shift-right: [w68] -> _
    shift-left: w18 -> [w82]
    shift-right: [w74] -> _
    shift-left: w18 -> [w81]
    shift-right: [w73] -> _
    shift-left: w18 -> [w80]
    i -> [w124]
    # "Is off"
    # "Is on"
    # "Ig off"
    # "Ig on"
    # "Is min"
    # "Is max"
    # "Ig min"
    # "Ig max"
    # "Id min"
    # "Id max"
    # "Id off"
    # "Id on"
    # "Pump status"
    # "Filepath and name"
    # "Pump status"
    # "Limit of command arguments (array columns). Raise if needed."
    # "Serial port data (string)"
    # "Serial port data (table)"
    # "Serial port data"
    # "For loop counter"
    # "<-----Equivalent to the 4155C \"Write\" subvi.----->"
    # "Headers"
    # "Save transfer curves in file."
    # "Filepath and name"
    # "Save time-dependent data."
    # "Use the time offset if your measurements do not start at t=0."
    # "Time for Imax, Imin, Ion, Ioff"
    # "Rest of elements of command"
    # "First element of command\n(case select)"
    n19 = Add(x=w124, y=1) -> (x+y=→"Line running":i32)
    n20 = Add(x=w129, y=1) -> (x+y=→"Total lines":i32)
    n21 = Index Array(array=w158, index=0 ("line index")) -> (element=w153:string)
    "Command running:" <- w153
    n22 = control-ref of="Interrupt run"() -> (w177:refnum<vi>)
    n23 = Spreadsheet String To Array(delimiter (Tab)=" ", format string="%s", spreadsheet string=w153, array type (2D Dbl)=string[] []) -> (array=w151:string[])
    n24 = Delete From Array(array=w151, index=0) -> (deleted portion=w100:string, array with subset deleted=w150:string[])  [unwired: 1 in]
    n25 = call "Elapsed Time"("Reset"="Reset", "Auto Reset"="Auto Reset") -> ("Elapsed Time (s)"=w160:dbl)  [unwired: 10 in, 7 out]
    n26 = case shown="2" "Time Units" {
      tunnel: ["-sec" "-min" "-h"] -> w161
      tunnel: [w191 w195 w198] -> w131
      tunnel: w160 -> [w191 w194 w199]
      frame 0, Default {
      }
      frame 1 {
        n27 = Divide(x=w194, y=60.0) -> (x/y=w195:dbl)
      }
      frame 2 {
        n28 = Divide(x=w199, y=3600.0) -> (x/y=w198:dbl)
      }
    }
    n29 = Add(x=w131, y="Time Offset") -> (x+y=w130:dbl)
    n30 = To Long Integer(number=w130) -> (32bit integer=w113:i32)
    "Elapsed Time" <- w113
    n31 = case shown="\"output\"" w100 {
      tunnel: w150 -> [w231 w264 w296 w424 w447 w584 w674 w822 w895 w922 w992 w1033 w1072 w1107 w1135 _ _ w1281 w1356 _ w1449 w1507 w1563 w1647 w1723 w1757]
      tunnel: w187 -> [w226 w260 w294 w431 w508 w592 w681 w829 w903 w940 w981 w1025 w1065 w1101 w1128 w1161 w1217 w1259 w1338 w1383 w1436 w1494 w1551 w1641 w1719 w1759]
      tunnel: w186 -> [w225 w259 w285 w402 w493 w561 w650 w800 w871 w941 w982 w1026 w1066 w1102 w1129 w1166 w1219 w1287 w1362 w1387 w1455 w1513 w1569 w1653 w1677 w1763]
      tunnel: w185 -> [w224 w258 w284 w401 w492 w560 w647 w799 w868 w942 w983 w1027 w1067 w1103 w1130 w1165 w1190 w1286 w1361 w1386 w1454 w1512 w1568 w1652 w1676 w1762]
      tunnel: w184 -> [w223 w257 w293 w427 w468 w588 w677 w825 w899 w950 w991 w1024 w1064 w1100 w1127 w1164 w1214 w1250 w1330 w1392 w1429 w1487 w1544 w1640 w1718 w1764]
      tunnel: w183 -> [w222 w256 w292 w429 w506 w590 w679 w827 w901 w949 w990 w1032 w1071 w1106 w1134 w1163 w1199 w1285 w1360 w1395 w1453 w1511 w1567 w1651 w1727 w1765]
      tunnel: w182 -> [w221 w255 w291 w428 w505 w589 w678 w826 w900 w948 w989 w1031 w1070 w1105 w1133 w1162 w1200 w1260 w1339 w1394 w1437 w1495 w1552 w1642 w1720 w1767]
      tunnel: [w225 w259 w283 w426 w503 w586 w676 w824 w897 w941 w982 w1026 w1066 w1102 w1129 w1166 w1219 w1251 w1312 w1385 w1430 w1488 w1545 w1593 w1679 w1763] -> w181
      tunnel: [w224 w258 w282 w425 w502 w585 w675 w823 w896 w942 w983 w1027 w1067 w1103 w1130 w1165 w1189 w1261 w1313 w1384 w1438 w1496 w1553 w1592 w1678 w1761] -> w112
      tunnel: [w223 w257 w293 w427 w464 w588 w677 w825 w899 w943 w984 w1024 w1064 w1100 w1127 w1164 w1214 w1250 w1330 w1392 w1429 w1487 w1544 w1640 w1718 w1764] -> w180
      tunnel: [w222 w256 w292 w429 w506 w590 w679 w827 w901 w949 w990 w1032 w1071 w1106 w1134 w1163 w1199 w1285 w1360 w1395 w1453 w1511 w1567 w1651 w1727 w1765] -> w179
      tunnel: [w221 w255 w291 w428 w505 w589 w678 w826 w900 w948 w989 w1031 w1070 w1105 w1133 w1162 w1200 w1260 w1339 w1394 w1437 w1495 w1552 w1642 w1720 w1767] -> w178
      tunnel: [w226 w260 w294 w431 w508 w592 w681 w829 w903 w940 w981 w1025 w1065 w1101 w1128 w1161 w1217 w1259 w1338 w1383 w1436 w1494 w1551 w1641 w1719 w1759] -> w66
      tunnel: w177 -> [_ _ _ w433 w512 w597 w684 w831 w907 _ _ _ _ _ _ _ _ w1256 w1335 _ w1435 w1493 w1550 w1613 w1695 _]
      tunnel: "Gate" -> [_ _ _ w411 w496 w571 w661 w809 w882 _ _ _ _ _ _ _ _ _ _ _ _ _ _ _ _ _]
      tunnel: "Drain 2" -> [_ _ _ w410 w495 w570 w660 w808 w881 _ _ _ _ _ _ _ _ _ _ _ _ _ _ _ _ _]
      tunnel: "Panel Controls" -> [_ _ _ _ _ w569 w659 w698 w880 _ _ _ _ _ _ _ _ _ _ _ _ _ _ _ _ _]
      tunnel: w173 -> [w220 w254 w290 w395 w486 w554 w645 w793 w866 w947 w988 _ w1063 w1099 w1126 w1160 w1201 w1246 w1326 w1388 w1425 w1483 w1540 w1636 w1714 w1768]
      tunnel: w172 -> [w219 w253 w289 w394 w485 w553 w644 w792 w865 w946 w987 w1030 _ w1090 w1132 w1159 w1202 w1247 w1327 w1389 w1426 w1484 w1541 w1637 w1715 w1769]
      tunnel: w171 -> [w218 w252 w288 w393 w484 w552 w643 w791 w864 w945 w986 w1029 w1069 w1104 _ w1158 w1203 w1248 w1328 w1390 w1427 w1485 w1542 w1638 w1716 w1770]
      tunnel: w170 -> [w217 w251 w287 w392 w483 w551 w646 w790 w867 w944 w985 w1028 w1068 _ w1131 w1157 w1204 w1249 w1329 w1391 w1428 w1486 w1543 w1639 w1717 w1771]
      tunnel: [w220 w254 w290 w395 w486 w554 w645 w793 w866 w947 w988 w1023 w1063 w1099 w1126 w1160 w1201 w1246 w1326 w1388 w1425 w1483 w1540 w1636 w1714 w1768] -> w169
      tunnel: [w219 w253 w289 w394 w485 w553 w644 w792 w865 w946 w987 w1030 w1055 w1090 w1132 w1159 w1202 w1247 w1327 w1389 w1426 w1484 w1541 w1637 w1715 w1769] -> w168
      tunnel: [w218 w252 w288 w393 w484 w552 w643 w791 w864 w945 w986 w1029 w1069 w1104 w1125 w1158 w1203 w1248 w1328 w1390 w1427 w1485 w1542 w1638 w1716 w1770] -> w167
      tunnel: [w217 w251 w287 w392 w483 w551 w646 w790 w867 w944 w985 w1028 w1068 w1091 w1131 w1157 w1204 w1249 w1329 w1391 w1428 w1486 w1543 w1639 w1717 w1771] -> w166
      tunnel: w165 -> [_ _ _ w387 w480 _ w639 w785 _ _ _ _ _ _ _ _ _ _ _ _ _ _ _ _ _ _]
      tunnel: w164 -> [_ _ _ w385 w479 _ _ _ _ _ _ _ _ _ _ _ _ _ _ _ _ _ _ _ _ _]
      tunnel: [w216 w247 w280 w317 w456 w541 w636 w716 w853 w939 w979 w1022 w1054 w1089 w1124 w1156 w1185 w1238 w1295 w1382 w1414 w1476 w1534 w1590 w1672 w1760] -> w78
      tunnel: w163 -> [w216 w247 w280 w382 w456 w541 w636 w781 w853 w939 w979 w1022 w1054 w1089 w1124 w1156 w1185 w1238 w1295 w1382 w1414 w1476 w1534 w1590 w1672 w1760]
      tunnel: w130 -> [_ _ _ w379 w453 w539 w634 w778 w850 _ _ _ _ _ _ _ w1183 w1236 w1308 _ w1411 w1473 w1531 w1587 w1668 _]
      tunnel: w161 -> [_ _ _ w376 w452 w537 w633 w775 w849 _ _ _ _ _ _ _ w1181 w1234 w1307 _ w1410 w1472 w1530 w1586 w1669 _]
      tunnel: w113 -> [_ _ _ w371 _ _ _ w770 _ _ _ _ _ _ _ _ _ _ _ _ _ _ _ _ _ _]
      tunnel: [w215 w246 w279 w325 w455 w540 w635 w724 w852 w938 w978 w1021 w1053 w1088 w1123 w1155 w1184 w1237 w1310 w1381 w1413 w1475 w1533 w1589 w1671 w1766] -> w114
      tunnel: w159 -> [w215 w246 w279 w375 w455 w540 w635 w774 w852 w938 w978 w1021 w1053 w1088 w1123 w1155 w1184 w1237 w1310 w1381 w1413 w1475 w1533 w1589 w1671 w1766]
      tunnel: [w214 w245 w278 w316 w451 w536 w632 w715 w848 w937 w977 w1020 w1052 w1087 w1122 w1154 w1180 w1233 w1294 w1380 w1409 w1471 w1529 w1585 w1667 w1755] -> w77
      tunnel: w135 -> [w214 w245 w278 w369 w451 w536 w632 w768 w848 w937 w977 w1020 w1052 w1087 w1122 w1154 w1180 w1233 w1294 w1380 w1409 w1471 w1529 w1585 w1667 w1755]
      tunnel: [w213 w244 w277 w362 w450 w535 w622 w761 w847 w936 w976 w1019 w1051 w1086 w1121 w1153 w1179 w1232 w1306 w1379 w1408 w1470 w1528 w1584 w1666 w1754] -> w108
      tunnel: w121 -> [w213 w244 w277 w362 w450 w535 w622 w761 w847 w936 w976 w1019 w1051 w1086 w1121 w1153 w1179 w1232 w1306 w1379 w1408 w1470 w1528 w1584 w1666 w1753]
      tunnel: [w212 w243 w276 w361 w449 w534 w621 w760 w846 w935 w975 w1018 w1050 w1085 w1120 w1152 w1178 w1231 w1305 w1378 w1407 w1469 w1527 w1583 w1665 w1739] -> w116
      tunnel: w115 -> [w212 w243 w276 w361 w449 w534 w621 w760 w846 w935 w975 w1018 w1050 w1085 w1120 w1152 w1178 w1231 w1305 w1378 w1407 w1469 w1527 w1583 w1665 w1739]
      tunnel: w113 -> [_ _ _ _ _ _ _ _ _ _ _ _ _ _ _ _ _ _ _ _ _ _ _ _ _ _]
      tunnel: [w211 w242 w275 w360 w448 w533 w620 w759 w845 w934 w974 w1017 w1049 w1084 w1119 w1151 w1177 w1230 w1304 w1377 w1406 w1468 w1526 w1582 w1664 w1738] -> w109
      tunnel: w111 -> [w211 w242 w275 w360 w448 w533 w620 w759 w845 w934 w974 w1017 w1049 w1084 w1119 w1151 w1177 w1230 w1304 w1377 w1406 w1468 w1526 w1582 w1664 w1738]
      tunnel: [w209 w240 w273 w310 w445 w531 w618 w709 w843 w932 w973 w1016 w1047 w1082 w1117 w1149 w1175 w1229 w1303 w1376 w1405 w1467 w1524 w1581 w1663 w1737] -> w71
      tunnel: w99 -> [w209 w240 w273 w356 w445 w531 w618 w755 w843 w932 w973 w1016 w1047 w1082 w1117 w1149 w1175 w1229 w1303 w1376 w1405 w1467 w1524 w1581 w1663 w1737]
      tunnel: [w210 w241 w274 w311 w446 w532 w619 w710 w844 w933 w972 w1015 w1048 w1083 w1118 w1150 w1176 w1228 w1302 w1375 w1404 w1466 w1525 w1580 w1662 w1736] -> w72
      tunnel: w98 -> [w210 w241 w274 w355 w446 w532 w619 w754 w844 w933 w972 w1015 w1048 w1083 w1118 w1150 w1176 w1228 w1302 w1375 w1404 w1466 w1525 w1580 w1662 w1736]
      tunnel: [w202 w233 w266 w315 w442 w529 w616 w714 w841 w925 w970 w1013 w1045 w1080 w1115 w1147 w1168 w1221 w1293 w1374 w1397 w1459 w1517 w1573 w1657 w1729] -> w76
      tunnel: w87 -> [w202 w233 w266 w345 w442 w529 w616 w744 w841 w925 w970 w1013 w1045 w1080 w1115 w1147 w1168 w1221 w1293 w1374 w1397 w1459 w1517 w1573 w1657 w1729]
      tunnel: [w201 w232 w265 w314 w443 w530 w617 w713 w842 w924 w971 w1014 w1046 w1081 w1116 w1148 w1167 w1220 w1292 w1373 w1396 w1458 w1516 w1572 w1656 w1728] -> w75
      tunnel: w86 -> [w201 w232 w265 w344 w443 w530 w617 w743 w842 w924 w971 w1014 w1046 w1081 w1116 w1148 w1167 w1220 w1292 w1373 w1396 w1458 w1516 w1572 w1656 w1728]
      tunnel: [w204 w235 w268 w320 w441 w527 w614 w719 w839 w930 w968 w1011 w1043 w1078 w1113 w1145 w1170 w1223 w1297 w1368 w1399 w1461 w1519 w1575 w1655 w1733] -> w69
      tunnel: w85 -> [w204 w235 w268 w341 w441 w527 w614 w740 w839 w930 w968 w1011 w1043 w1078 w1113 w1145 w1170 w1223 w1297 w1368 w1399 w1461 w1519 w1575 w1655 w1733]
      tunnel: [w203 w234 w267 w318 w444 w528 w615 w717 w840 w931 w969 w1012 w1044 w1079 w1114 w1146 w1169 w1222 w1296 w1367 w1398 w1460 w1518 w1574 w1654 w1732] -> w79
      tunnel: w84 -> [w203 w234 w267 w340 w444 w528 w615 w739 w840 w931 w969 w1012 w1044 w1079 w1114 w1146 w1169 w1222 w1296 w1367 w1398 w1460 w1518 w1574 w1654 w1732]
      tunnel: [w206 w237 w270 w309 w440 w525 w612 w708 w837 w928 w966 w1009 w1041 w1076 w1111 w1143 w1172 w1225 w1299 w1370 w1401 w1463 w1521 w1577 w1659 w1735] -> w70
      tunnel: w83 -> [w206 w237 w270 w337 w440 w525 w612 w736 w837 w928 w966 w1009 w1041 w1076 w1111 w1143 w1172 w1225 w1299 w1370 w1401 w1463 w1521 w1577 w1659 w1735]
      tunnel: [w205 w236 w269 w308 w439 w526 w613 w707 w838 w929 w967 w1010 w1042 w1077 w1112 w1144 w1171 w1224 w1298 w1369 w1400 w1462 w1520 w1576 w1658 w1734] -> w68
      tunnel: w82 -> [w205 w236 w269 w336 w439 w526 w613 w735 w838 w929 w967 w1010 w1042 w1077 w1112 w1144 w1171 w1224 w1298 w1369 w1400 w1462 w1520 w1576 w1658 w1734]
      tunnel: [w208 w239 w272 w313 w438 w523 w610 w712 w835 w926 w964 w1007 w1039 w1074 w1109 w1141 w1174 w1227 w1301 w1372 w1403 w1465 w1523 w1579 w1661 w1731] -> w74
      tunnel: w81 -> [w208 w239 w272 w333 w438 w523 w610 w732 w835 w926 w964 w1007 w1039 w1074 w1109 w1141 w1174 w1227 w1301 w1372 w1403 w1465 w1523 w1579 w1661 w1731]
      tunnel: [w207 w238 w271 w312 w437 w524 w611 w711 w836 w927 w965 w1008 w1040 w1075 w1110 w1142 w1173 w1226 w1300 w1371 w1402 w1464 w1522 w1578 w1660 w1730] -> w73
      tunnel: w80 -> [w207 w238 w271 w332 w437 w524 w611 w731 w836 w927 w965 w1008 w1040 w1075 w1110 w1142 w1173 w1226 w1300 w1371 w1402 w1464 w1522 w1578 w1660 w1730]
      frame "wait" {
        n32 = Index Array(array=w231, index=0 ("Index")) -> (element=w229:string)
        n33 = Decimal String To Number(string=w229, default (0L)=u32 0) -> (number=w228:u32)  [unwired: 1 in, 1 out]
        n34 = Wait (ms)(milliseconds to wait=w228) -> ()  [unwired: 1 out]
      }
      frame "wait-min" {
        n35 = Index Array(array=w264, index=0 ("Index")) -> (element=w262:string)
        n36 = Decimal String To Number(string=w262, default (0L)=u32 0) -> (number=w250:u32)  [unwired: 1 in, 1 out]
        n37 = Multiply(x=w250, y=u32 60000) -> (x*y=w249:u32)
        n38 = Wait (ms)(milliseconds to wait=w249) -> ()  [unwired: 1 out]
      }
      frame "standby" {
        n39 = Index Array(array=w296, index=0 ("Index")) -> (element=w286:string)
        n40 = case shown="\"off\", Default" w286 {
          tunnel: [":PAGE:SCON:STAN 0" ":PAGE:SCON:STAN 1"] -> w281
          frame "off", Default {
          }
          frame "on" {
          }
        }
        n41 = VISA Write(VISA resource name=w285, write buffer=w281, error in (no error)=w284) -> (VISA resource name out=w283:refnum<visa-resource-name>, error out=w282:errorcluster)  [unwired: 1 out]
      }
      frame "transfer" {
        # "Adjusts graph colors."
        # "Adjusts graph colors."
        # "Is off"
        # "Is on"
        # "Ion will be the middle element of the array. The calculation of the index is done only once, since Is, Id, and Ig have the same dimensions."
        # "Ig off"
        # "Ig on"
        # "Is min"
        # "Is max"
        # "Ig min"
        # "Ig max"
        # "abs(Ig)"
        # "abs(Is)"
        # "Id min"
        # "Id max"
        # "Y1: Is\nY2: Id\nY3: Ig"
        # "abs(Id)"
        # "Adjusts graph colors."
        # "Adjusts graph colors."
        # "Id off"
        # "Id on"
        # "Adjusts graph colors."
        # "Time array"
        n42 = Delete From Array(array=w424, index=0 ("Index")) -> (deleted portion=w422:string, array with subset deleted=w421:string[])  [unwired: 1 in]
        n43 = Bundle By Name(cluster=w385, "Emergency Stop"=w433) -> (w386:T3)
        n44 = Number To Decimal String(number=w379) -> (decimal integer string=w378:string)  [unwired: 1 in]
        n45 = case shown="\"d\", Default" w422 {
          tunnel: [w435 w436] -> w420
          frame "s" {
            w435 = u16 0 items=["Single", "Double"] ("sweep mode")
          }
          frame "d", Default {
            w436 = u16 1 items=["Single", "Double"] ("sweep mode")
          }
        }
        n46 = Fract/Exp String To Number(string=w421) -> (number=w406:dbl[])  [unwired: 3 in, 1 out]
        n47 = Concatenate Strings(w431, "-transfer-" ("Prefix"), w378, w376, ".txt" ("Suffix (transfer)")) -> (w432:string)
        n48 = VISA Write(VISA resource name=w402, write buffer=":PAGE:CHAN:MODE SWE;" ("write buffer (\"\")"), error in (no error)=w401) -> (VISA resource name out=w399:refnum<visa-resource-name>, error out=w400:errorcluster)  [unwired: 1 out]
        n49 = String To Path(string=w432) -> (path=w430:path)
        n50 = Index Array(array=w406, index #1=0 ("Index")) -> (element #1=w419:dbl, element #2=w418:dbl, element #3=w417:dbl)  [unwired: 2 in]
        n51 = Delete From Array(array=w406, length=3 ("Length"), index=0 ("Index")) -> (array with subset deleted=w404:dbl[])  [unwired: 1 out]
        n52 = Build Array (concatenate)(w375, w371) -> (w325:i32[])
        n53 = Bundle By Name(cluster=w411, "Gate Start"=w419, "Gate Stop"=w418, "Gate Step (linear only)"=w417, "Gate Compliance"=w428, "Range mode"=w395, "Range"=w394) -> (w396:T6)
        n54 = control-ref of="Imax vs time"() -> (w354:refnum<vi>)
        n55 = control-ref of="Imin vs time"() -> (w353:refnum<vi>)
        n56 = control-ref of="Ion vs time"() -> (w322:refnum<vi>)
        n57 = control-ref of="Ioff vs time"() -> (w321:refnum<vi>)
        n58 = control-ref of="I vs Vg"() -> (w380:refnum<vi>)
        n59 = Index Array(array=w404, index #1=0 ("Index")) -> (element #1=w414:dbl, element #2=w413:dbl, element #3=w412:dbl)  [unwired: 2 in]
        n60 = call <vilib>:"compatOverwrite.vi"("overwrite (F)"=TRUE) -> ("overwrite?"=w384:T8)
        n61 = Bundle By Name(cluster=w410, "Drain Start"=w414, "Drain Stop"=w413, "Drain Step"=w412, "Drain Compliance"=w429, "Range mode"=w393, "Range"=w392) -> (w397:T7)
        n62 = call "4155C Transfer.vi"("VISA resource name in"=w399, "Gate"=w396, "Drain"=w397, "Timings"=w427, "error in (no error)"=w400, "SMU4"=w387, "sweep mode"=w420, "Panel Controls"=w386) -> ("VG"=w383:dbl[], "Outparams"=w391:T9, "VISA Resource Name out"=w426:refnum<visa-resource-name>, "IS"=w350:dbl[], "ID"=w352:dbl[], "IG"=w349:dbl[], "error out"=w372:errorcluster, "SMU4"=w388:dbl[])  [unwired: 12 in]
        n63 = Unbundle By Name(w391) -> ("V2 Step"=w390:dbl, "V2 Start"=w389:dbl, "Number of points"=w319:i32)
        n64 = Absolute Value(x=w350) -> (abs(x)=w335:dbl[])
        n65 = Absolute Value(x=w352) -> (abs(x)=w351:dbl[])
        n66 = Absolute Value(x=w349) -> (abs(x)=w338:dbl[])
        n67 = Array Size(array=w351) -> (size(s)=w359:i32)
        n68 = Divide(x=w359, y=2) -> (x/y=w302:dbl)
        n69 = Subtract(x=w302, y=1) -> (x-y=w301:dbl)
        n70 = Array Max & Min(array=w335) -> (max value=w342:dbl, min value=w343:dbl)  [unwired: 2 out]
        n71 = Array Max & Min(array=w351) -> (max value=w381:dbl, min value=w348:dbl)  [unwired: 2 out]
        n72 = Array Max & Min(array=w338) -> (max value=w347:dbl, min value=w346:dbl)  [unwired: 2 out]
        n73 = call "4155C Split array.vi"("Number of VAR2 steps"=w319, "Y2 data in"=w352, "X data in"=w383, "Y1 data in"=w350, "Y3 data in"=w349, "error in (no error)"=w372) -> ("Array of clusters"=w374:cluster{"Y data in":dbl[], "X data in":dbl[]}[], "error out"=w307:errorcluster)  [unwired: 1 in]
        n74 = Index Array(array=w335, index=w301) -> (element=w326:dbl)
        n75 = Index Array(array=w335, index=0) -> (element=w327:dbl)
        n76 = Index Array(array=w351, index=w301) -> (element=w328:dbl)
        n77 = Index Array(array=w351, index=0) -> (element=w329:dbl)
        n78 = Index Array(array=w338, index=w301) -> (element=w331:dbl)
        n79 = Index Array(array=w338, index=0) -> (element=w330:dbl)
        n80 = local write "Ig max"(w347) -> ()
        n81 = local write "Ig min"(w346) -> ()
        n82 = local write "Is max"(w342) -> ()
        n83 = local write "Is min"(w343) -> ()
        n84 = local write "Id max"(w381) -> ()
        n85 = local write "Id min"(w348) -> ()
        n86 = local write "I vs Vg"(w374) -> ()
        n87 = Build Array (concatenate)(w341, w342) -> (w320:dbl[])
        n88 = Build Array (concatenate)(w340, w343) -> (w318:dbl[])
        n89 = local write "Is off"(w327) -> ()
        n90 = local write "Is on"(w326) -> ()
        n91 = Build Array (concatenate)(w382, w381) -> (w317:dbl[])
        n92 = Build Array (concatenate)(w369, w348) -> (w316:dbl[])
        n93 = Build Array (concatenate)(w345, w347) -> (w315:dbl[])
        n94 = Build Array (concatenate)(w344, w346) -> (w314:dbl[])
        n95 = Build Array (concatenate)(w333, w326) -> (w313:dbl[])
        n96 = Build Array (concatenate)(w332, w327) -> (w312:dbl[])
        n97 = Build Array (concatenate)(w355, w328) -> (w311:dbl[])
        n98 = Build Array (concatenate)(w356, w329) -> (w310:dbl[])
        n99 = Build Array (concatenate)(w337, w331) -> (w309:dbl[])
        n100 = Build Array (concatenate)(w336, w330) -> (w308:dbl[])
        n101 = local write "Ig off"(w330) -> ()
        n102 = local write "Ig on"(w331) -> ()
        n103 = local write "Id off"(w329) -> ()
        n104 = local write "Id on"(w328) -> ()
        n105 = call "4155C Split array.vi"("Number of VAR2 steps"=w319, "Y2 data in"=w311, "X data in"=w325, "Y1 data in"=w313, "Y3 data in"=w309, "error in (no error)"=w307) -> ("Array of clusters"=w323:cluster{"Y data in":dbl[], "X data in":dbl[]}[], "error out"=w306:errorcluster)  [unwired: 1 in]
        n106 = call "4155C Split array.vi"("Number of VAR2 steps"=w319, "Y2 data in"=w310, "X data in"=w325, "Y1 data in"=w312, "Y3 data in"=w308, "error in (no error)"=w306) -> ("Array of clusters"=w324:cluster{"Y data in":dbl[], "X data in":dbl[]}[], "error out"=w305:errorcluster)  [unwired: 1 in]
        n107 = call "4155C Split array.vi"("Number of VAR2 steps"=w319, "Y2 data in"=w317, "X data in"=w325, "Y1 data in"=w320, "Y3 data in"=w315, "error in (no error)"=w305) -> ("Array of clusters"=w373:cluster{"Y data in":dbl[], "X data in":dbl[]}[], "error out"=w304:errorcluster)  [unwired: 1 in]
        n108 = call "4155C Split array.vi"("Number of VAR2 steps"=w319, "Y2 data in"=w316, "X data in"=w325, "Y1 data in"=w318, "Y3 data in"=w314, "error in (no error)"=w304) -> ("Array of clusters"=w370:cluster{"Y data in":dbl[], "X data in":dbl[]}[], "error out"=w303:errorcluster)  [unwired: 1 in]
        n109 = Open/Create/Replace File(file path (use dialog)=w430, error in=w303, operation (0:open)=w384) -> (refnum out=w367:refnum<file>, error out=w365:errorcluster)  [unwired: 3 in, 1 out]
        n110 = call "4155C Make Big 2d array.vi"("1D Var1"=w383, "1d IS"=w350, "1d ID"=w352, "1d IG"=w349, "1d SMU4"=w388, "SMU4"=w387, "VAR2 START"=w389, "Number of VAR2 steps"=w319, "VAR2 STEP"=w390, "VAR1 Name"="Vg", "Decimal places in header"=i8 1, "VAR2 Name"="Vd") -> ("Header array"=w368:string[], "Data array"=w366:dbl[][])  [unwired: 14 in]
        n111 = local write "Imax vs time"(w373) -> ()
        n112 = local write "Imin vs time"(w370) -> ()
        n113 = local write "Ion vs time"(w323) -> ()
        n114 = local write "Ioff vs time"(w324) -> ()
        n115 = call "4155C Config Chart Colours.vi"("Numeric"=w319, "XY Graph 2"=w354) -> ()  [unwired: 6 in]
        n116 = call "4155C Config Chart Colours.vi"("Numeric"=w319, "XY Graph 2"=w353) -> ()  [unwired: 6 in]
        n117 = call "4155C Config Chart Colours.vi"("Numeric"=w319, "XY Graph 2"=w322) -> ()  [unwired: 6 in]
        n118 = call "4155C Config Chart Colours.vi"("Numeric"=w319, "XY Graph 2"=w321) -> ()  [unwired: 6 in]
        n119 = call "4155C Config Chart Colours.vi"("Numeric"=w319, "XY Graph 2"=w380) -> ()  [unwired: 6 in]
        n120 = call "4155C Write array to file.vi"("Byte Stream File Refnum"=w367, "Header"=w368, "Data Array"=w366, "error in (no error)"=w365) -> ("dup refnum"=w364:refnum<file>, "error out"=w363:errorcluster)  [unwired: 1 in]
        n121 = Close File(refnum=w364, error in=w363) -> (error out=w425:errorcluster)  [unwired: 1 out]
      }
      frame "pulsedstressV" {
        w462 = 0
        n122 = Number To Decimal String(number=w453) -> (decimal integer string=w509:string)  [unwired: 1 in]
        n123 = Delete From Array(array=w447, index=0 ("Index")) -> (deleted portion=w500:string, array with subset deleted=w499:string[])  [unwired: 1 in]
        n124 = Bundle By Name(cluster=w479, "Emergency Stop"=w512) -> (w481:T3)
        n125 = VISA Write(VISA resource name=w493, write buffer=":PAGE:CHAN:MODE SWE;" ("write buffer (\"\")"), error in (no error)=w492) -> (VISA resource name out=w490:refnum<visa-resource-name>, error out=w491:errorcluster)  [unwired: 1 out]
        n126 = Concatenate Strings(w508, "-pulsedstressV-" ("Substring"), w509, w452, ".txt" ("Substring")) -> (w511:string)
        n127 = case shown="\"d\", Default" w500 {
          tunnel: [w521 w522] -> w498
          frame "s" {
            w521 = u16 0 items=["Single", "Double"] ("sweep mode")
          }
          frame "d", Default {
            w522 = u16 1 items=["Single", "Double"] ("sweep mode")
          }
        }
        n128 = Fract/Exp String To Number(string=w499) -> (number=w494:dbl[])  [unwired: 3 in, 1 out]
        n129 = String To Path(string=w511) -> (path=w507:path)
        n130 = Index Array(array=w494, index #1=0 ("Index")) -> (element #1=w471:dbl, element #2=w470:dbl, element #3=w467:dbl, element #4=w466:dbl, element #5=w465:dbl, element #6=w469:dbl)  [unwired: 5 in]
        n131 = Bundle By Name(cluster=w468, "Pulse period"=w466, "Base voltage"=w467, "Pulse width"=w465) -> (w464:T5)
        n132 = Unbundle By Name(w464) -> ("Pulse period"=w472:dbl)
        n133 = Bundle By Name(cluster=w496, "Gate Start"=w470, "Gate Stop"=w471, "Gate Step (linear only)"=0, "Gate Compliance"=w505, "Range mode"=w486, "Range"=w485) -> (w487:T6)
        n134 = call <vilib>:"compatOverwrite.vi"("overwrite (F)"=TRUE) -> ("overwrite?"=w457:T8)
        n135 = Bundle By Name(cluster=w495, "Drain Start"=w469, "Drain Stop"=w462, "Drain Step"=w462, "Drain Compliance"=w506, "Range mode"=w484, "Range"=w483) -> (w488:T7)
        n136 = call "4155C PulsedStressV.vi"("VISA resource name in"=w490, "sweep mode"=w498, "Panel Controls"=w481, "Gate"=w487, "Drain"=w488, "Timings"=w464, "error in (no error)"=w491, "SMU4"=w480) -> ("VISA Resource Name out"=w503:refnum<visa-resource-name>, "ID"=w460:dbl[], "IG"=w458:dbl[], "Outparams"=w482:T9, "error out"=w504:errorcluster)  [unwired: 3 in]
        n137 = Unbundle By Name(w482) -> ("Number of points"=w459:i32)  [unwired: 2 out]
        n138 = for {
          N: w459 -> [_]
          tunnel: [w518] -> w461 mode=indexing
          tunnel: w472 -> [w520]
          i -> [w519]
          n139 = Multiply(x=w520, y=w519) -> (x*y=w518:dbl)
        }
        n140 = Insert Into Array(array=dbl[][] [] ("Input Array"), new element=w461) -> (w473:dbl[][])  [unwired: 2 in]
        n141 = Insert Into Array(array=w473, new element=w460) -> (w478:dbl[][])  [unwired: 2 in]
        n142 = Insert Into Array(array=w478, new element=w458) -> (w477:dbl[][])  [unwired: 2 in]
        n143 = Transpose 2D Array(2D array=w477) -> (transposed array=w476:dbl[][])
        n144 = Open/Create/Replace File(file path (use dialog)=w507, error in=w504, operation (0:open)=w457) -> (refnum out=w515:refnum<file>, error out=w516:errorcluster)  [unwired: 3 in, 1 out]
        n145 = call "4155C Write array to file.vi"("Byte Stream File Refnum"=w515, "Header"=string[] ["Time /s", "Id /A", "Ig /A"], "Data Array"=w476, "error in (no error)"=w516) -> ("dup refnum"=w513:refnum<file>, "error out"=w514:errorcluster)  [unwired: 1 in]
        n146 = Close File(refnum=w513, error in=w514) -> (error out=w502:errorcluster)  [unwired: 1 out]
      }
      frame "transfer-fpp" {
        n147 = Number To Decimal String(number=w539) -> (decimal integer string=w593:string)  [unwired: 1 in]
        n148 = Bundle By Name(cluster=w569, "Emergency Stop"=w597) -> (w605:T2)
        n149 = Delete From Array(array=w584, index=0 ("Index")) -> (deleted portion=w582:string, array with subset deleted=w581:string[])  [unwired: 1 in]
        n150 = Concatenate Strings(w592, "-transferfpp-" ("Substring"), w593, w537, ".txt" ("Substring")) -> (w595:string)
        n151 = VISA Write(VISA resource name=w561, write buffer=":PAGE:CHAN:MODE SWE;" ("write buffer (\"\")"), error in (no error)=w560) -> (VISA resource name out=w558:refnum<visa-resource-name>, error out=w559:errorcluster)  [unwired: 1 out]
        n152 = case shown="\"d\", Default" w582 {
          tunnel: [w606 w607] -> w580
          frame "s" {
            w606 = u16 0 items=["Single", "Double"] ("sweep mode")
          }
          frame "d", Default {
            w607 = u16 1 items=["Single", "Double"] ("sweep mode")
          }
        }
        n153 = Fract/Exp String To Number(string=w581) -> (number=w565:dbl[])  [unwired: 3 in, 1 out]
        n154 = String To Path(string=w595) -> (path=w591:path)
        n155 = Index Array(array=w565, index #1=0 ("Index")) -> (element #1=w579:dbl, element #2=w578:dbl, element #3=w577:dbl)  [unwired: 2 in]
        n156 = Delete From Array(array=w565, length=3 ("Length"), index=0 ("Index")) -> (array with subset deleted=w563:dbl[])  [unwired: 1 out]
        n157 = Bundle By Name(cluster=w571, "Gate Start"=w579, "Gate Stop"=w578, "Gate Step (linear only)"=w577, "Gate Compliance"=w589, "Range mode"=w554, "Range"=w553) -> (w555:T6)
        n158 = Index Array(array=w563, index #1=0 ("Index")) -> (element #1=w574:dbl, element #2=w573:dbl, element #3=w572:dbl)  [unwired: 2 in]
        n159 = call <vilib>:"compatOverwrite.vi"("overwrite (F)"=TRUE) -> ("overwrite?"=w542:T8)
        n160 = Bundle By Name(cluster=w570, "Drain Start"=w574, "Drain Stop"=w573, "Drain Step"=w572, "Drain Compliance"=w590, "Range mode"=w552, "Range"=w551) -> (w556:T7)
        n161 = call "4155C Transfer-FPP.vi"("VISA resource name in"=w558, "Gate"=w555, "Drain"=w556, "Timings"=w588, "error in (no error)"=w559, "sweep mode"=w580, "Panel Controls"=w605) -> ("VG"=w596:dbl[], "Outparams"=w550:T9, "VISA Resource Name out"=w586:refnum<visa-resource-name>, "Vprobe2"=w546:dbl[], "ID"=w545:dbl[], "IG"=w544:dbl[], "Vprobe1"=w543:dbl[], "error out"=w587:errorcluster)  [unwired: 13 in]
        n162 = Unbundle By Name(w550) -> ("V2 Step"=w549:dbl, "V2 Start"=w548:dbl, "Number of points"=w547:i32)
        n163 = Open/Create/Replace File(file path (use dialog)=w591, error in=w587, operation (0:open)=w542) -> (refnum out=w602:refnum<file>, error out=w603:errorcluster)  [unwired: 3 in, 1 out]
        n164 = call "4155C Make Big 2d array FPP.vi"("1D Var1"=w596, "1d ID"=w545, "1d Vp2"=w546, "1d IG"=w544, "1d Vp1"=w543, "VAR2 START"=w548, "Number of VAR2 steps"=w547, "VAR2 STEP"=w549, "VAR1 Name"="Vg", "Decimal places in header"=i8 1, "VAR2 Name"="Vd") -> ("Header array"=w598:string[], "Data array"=w599:dbl[][])  [unwired: 15 in]
        n165 = call "4155C Write array to file.vi"("Byte Stream File Refnum"=w602, "Header"=w598, "Data Array"=w599, "error in (no error)"=w603) -> ("dup refnum"=w600:refnum<file>, "error out"=w601:errorcluster)  [unwired: 1 in]
        n166 = Close File(refnum=w600, error in=w601) -> (error out=w585:errorcluster)  [unwired: 1 out]
      }
      frame "output" {
        n167 = Number To Decimal String(number=w634) -> (decimal integer string=w682:string)  [unwired: 1 in]
        n168 = Bundle By Name(cluster=w659, "Emergency Stop"=w684) -> (w694:T2)
        n169 = Delete From Array(array=w674, index=0 ("Index")) -> (deleted portion=w672:string, array with subset deleted=w671:string[])  [unwired: 1 in]
        n170 = Concatenate Strings(w681, "-output-" ("Substring"), w682, w633, ".txt" ("Suffix (output)")) -> (w683:string)
        n171 = VISA Write(VISA resource name=w650, write buffer=":PAGE:CHAN:MODE SWE;" ("write buffer (\"\")"), error in (no error)=w647) -> (VISA resource name out=w649:refnum<visa-resource-name>, error out=w648:errorcluster)  [unwired: 1 out]
        n172 = case shown="\"d\", Default" w672 {
          tunnel: [w695 w696] -> w670
          frame "s" {
            w695 = u16 0 items=["Single", "Double"] ("sweep mode")
          }
          frame "d", Default {
            w696 = u16 1 items=["Single", "Double"] ("sweep mode")
          }
        }
        n173 = Fract/Exp String To Number(string=w671) -> (number=w653:dbl[])  [unwired: 3 in, 1 out]
        n174 = String To Path(string=w683) -> (path=w680:path)
        n175 = Index Array(array=w653, index #1=0 ("Index")) -> (element #1=w669:dbl, element #2=w668:dbl, element #3=w667:dbl)  [unwired: 2 in]
        n176 = Delete From Array(array=w653, length=3 ("Length"), index=0 ("Index")) -> (array with subset deleted=w652:dbl[])  [unwired: 1 out]
        n177 = control-ref of="I vs Vd"() -> (w624:refnum<vi>)
        n178 = Bundle By Name(cluster=w661, "Gate Start"=w669, "Gate Stop"=w668, "Gate Step (linear only)"=w667, "Gate Compliance"=w678, "Range mode"=w645, "Range"=w644) -> (w693:T6)
        n179 = Index Array(array=w652, index #1=0 ("Index")) -> (element #1=w664:dbl, element #2=w663:dbl, element #3=w662:dbl)  [unwired: 2 in]
        n180 = call <vilib>:"compatOverwrite.vi"("overwrite (F)"=TRUE) -> ("overwrite?"=w637:T8)
        n181 = Bundle By Name(cluster=w660, "Drain Start"=w664, "Drain Stop"=w663, "Drain Step"=w662, "Drain Compliance"=w679, "Range mode"=w643, "Range"=w646) -> (w692:T7)
        n182 = call "4155C Output.vi"("VISA resource name in"=w649, "Gate"=w693, "Drain"=w692, "Timings"=w677, "error in (no error)"=w648, "SMU4"=w639, "sweep mode"=w670, "Panel controls"=w694) -> ("VD"=w631:dbl[], "Outparams"=w641:T9, "VISA Resource Name out"=w676:refnum<visa-resource-name>, "IS"=w630:dbl[], "ID"=w629:dbl[], "IG"=w628:dbl[], "error out"=w626:errorcluster, "SMU4"=w638:dbl[])  [unwired: 12 in]
        n183 = Unbundle By Name(w641) -> ("V2 Step"=w642:dbl, "V2 Start"=w640:dbl, "Number of points"=w623:i32)
        n184 = call "4155C Split array.vi"("Number of VAR2 steps"=w623, "Y2 data in"=w629, "X data in"=w631, "Y1 data in"=w630, "Y3 data in"=w628, "error in (no error)"=w626) -> ("Array of clusters"=w627:cluster{"Y data in":dbl[], "X data in":dbl[]}[], "error out"=w625:errorcluster)  [unwired: 1 in]
        n185 = local write "I vs Vd"(w627) -> ()
        n186 = call "4155C Config Chart Colours.vi"("Numeric"=w623, "XY Graph 2"=w624) -> ()  [unwired: 6 in]
        n187 = Open/Create/Replace File(file path (use dialog)=w680, error in=w625, operation (0:open)=w637) -> (refnum out=w689:refnum<file>, error out=w690:errorcluster)  [unwired: 3 in, 1 out]
        n188 = call "4155C Make Big 2d array.vi"("1D Var1"=w631, "1d IS"=w630, "1d ID"=w629, "1d IG"=w628, "1d SMU4"=w638, "SMU4"=w639, "VAR2 START"=w640, "Number of VAR2 steps"=w623, "VAR2 STEP"=w642, "VAR1 Name"="Vd", "Decimal places in header"=i8 1, "VAR2 Name"="Vg") -> ("Header array"=w685:string[], "Data array"=w686:dbl[][])  [unwired: 14 in]
        n189 = call "4155C Write array to file.vi"("Byte Stream File Refnum"=w689, "Header"=w685, "Data Array"=w686, "error in (no error)"=w690) -> ("dup refnum"=w687:refnum<file>, "error out"=w688:errorcluster)  [unwired: 1 in]
        n190 = Close File(refnum=w687, error in=w688) -> (error out=w675:errorcluster)  [unwired: 1 out]
      }
      frame "output2" {
        # "Adjusts graph colors."
        # "Adjusts graph colors."
        # "Is off"
        # "Is on"
        # "Ion will be the middle element of the array. The calculation of the index is done only once, since Is, Id, and Ig have the same dimensions."
        # "Ig off"
        # "Ig on"
        # "Is min"
        # "Is max"
        # "Ig min"
        # "Ig max"
        # "abs(Ig)"
        # "abs(Is)"
        # "Id min"
        # "Id max"
        # "Y1: Is\nY2: Id\nY3: Ig"
        # "abs(Id)"
        # "Adjusts graph colors."
        # "Adjusts graph colors."
        # "Id off"
        # "Id on"
        # "Adjusts graph colors."
        # "Time array"
        n191 = Delete From Array(array=w822, index=0 ("Index")) -> (deleted portion=w820:string, array with subset deleted=w819:string[])  [unwired: 1 in]
        n192 = Bundle By Name(cluster=w698, "Emergency Stop"=w831) -> (w784:T2)
        n193 = Number To Decimal String(number=w778) -> (decimal integer string=w777:string)  [unwired: 1 in]
        n194 = case shown="\"d\", Default" w820 {
          tunnel: [w833 w834] -> w818
          frame "s" {
            w833 = u16 0 items=["Single", "Double"] ("sweep mode")
          }
          frame "d", Default {
            w834 = u16 1 items=["Single", "Double"] ("sweep mode")
          }
        }
        n195 = Fract/Exp String To Number(string=w819) -> (number=w804:dbl[])  [unwired: 3 in, 1 out]
        n196 = Concatenate Strings(w829, "-output-" ("Substring"), w777, w775, ".txt" ("Suffix (transfer)")) -> (w830:string)
        n197 = VISA Write(VISA resource name=w800, write buffer=":PAGE:CHAN:MODE SWE;" ("write buffer (\"\")"), error in (no error)=w799) -> (VISA resource name out=w797:refnum<visa-resource-name>, error out=w798:errorcluster)  [unwired: 1 out]
        n198 = String To Path(string=w830) -> (path=w828:path)
        n199 = Index Array(array=w804, index #1=0 ("Index")) -> (element #1=w817:dbl, element #2=w816:dbl, element #3=w815:dbl)  [unwired: 2 in]
        n200 = Delete From Array(array=w804, length=3 ("Length"), index=0 ("Index")) -> (array with subset deleted=w802:dbl[])  [unwired: 1 out]
        n201 = Build Array (concatenate)(w774, w770) -> (w724:i32[])
        n202 = Bundle By Name(cluster=w809, "Gate Start"=w817, "Gate Stop"=w816, "Gate Step (linear only)"=w815, "Gate Compliance"=w826, "Range mode"=w793, "Range"=w792) -> (w794:T6)
        n203 = control-ref of="Imax vs time"() -> (w753:refnum<vi>)
        n204 = control-ref of="Imin vs time"() -> (w752:refnum<vi>)
        n205 = control-ref of="Ion vs time"() -> (w721:refnum<vi>)
        n206 = control-ref of="Ioff vs time"() -> (w720:refnum<vi>)
        n207 = control-ref of="I vs Vg"() -> (w779:refnum<vi>)
        n208 = Index Array(array=w802, index #1=0 ("Index")) -> (element #1=w812:dbl, element #2=w811:dbl, element #3=w810:dbl)  [unwired: 2 in]
        n209 = call <vilib>:"compatOverwrite.vi"("overwrite (F)"=TRUE) -> ("overwrite?"=w783:T8)
        n210 = Bundle By Name(cluster=w808, "Drain Start"=w812, "Drain Stop"=w811, "Drain Step"=w810, "Drain Compliance"=w827, "Range mode"=w791, "Range"=w790) -> (w795:T7)
        n211 = call "4155C Output.vi"("VISA resource name in"=w797, "Gate"=w794, "Drain"=w795, "Timings"=w825, "error in (no error)"=w798, "SMU4"=w785, "sweep mode"=w818, "Panel controls"=w784) -> ("VD"=w782:dbl[], "Outparams"=w789:T9, "VISA Resource Name out"=w824:refnum<visa-resource-name>, "IS"=w749:dbl[], "ID"=w751:dbl[], "IG"=w748:dbl[], "error out"=w771:errorcluster, "SMU4"=w786:dbl[])  [unwired: 12 in]
        n212 = Unbundle By Name(w789) -> ("V2 Step"=w788:dbl, "V2 Start"=w787:dbl, "Number of points"=w718:i32)
        n213 = Absolute Value(x=w749) -> (abs(x)=w734:dbl[])
        n214 = Absolute Value(x=w751) -> (abs(x)=w750:dbl[])
        n215 = Absolute Value(x=w748) -> (abs(x)=w737:dbl[])
        n216 = Array Size(array=w750) -> (size(s)=w758:i32)
        n217 = Divide(x=w758, y=2) -> (x/y=w701:dbl)
        n218 = Subtract(x=w701, y=1) -> (x-y=w700:dbl)
        n219 = Array Max & Min(array=w734) -> (max value=w741:dbl, min value=w742:dbl)  [unwired: 2 out]
        n220 = Array Max & Min(array=w750) -> (max value=w780:dbl, min value=w747:dbl)  [unwired: 2 out]
        n221 = Array Max & Min(array=w737) -> (max value=w746:dbl, min value=w745:dbl)  [unwired: 2 out]
        n222 = call "4155C Split array.vi"("Number of VAR2 steps"=w718, "Y2 data in"=w751, "X data in"=w782, "Y1 data in"=w749, "Y3 data in"=w748, "error in (no error)"=w771) -> ("Array of clusters"=w773:cluster{"Y data in":dbl[], "X data in":dbl[]}[], "error out"=w706:errorcluster)  [unwired: 1 in]
        n223 = Index Array(array=w734, index=w700) -> (element=w725:dbl)
        n224 = Index Array(array=w734, index=0) -> (element=w726:dbl)
        n225 = Index Array(array=w750, index=w700) -> (element=w727:dbl)
        n226 = Index Array(array=w750, index=0) -> (element=w728:dbl)
        n227 = Index Array(array=w737, index=w700) -> (element=w730:dbl)
        n228 = Index Array(array=w737, index=0) -> (element=w729:dbl)
        n229 = local write "Ig max"(w746) -> ()
        n230 = local write "Ig min"(w745) -> ()
        n231 = local write "Is max"(w741) -> ()
        n232 = local write "Is min"(w742) -> ()
        n233 = local write "Id max"(w780) -> ()
        n234 = local write "Id min"(w747) -> ()
        n235 = local write "I vs Vd"(w773) -> ()
        n236 = Build Array (concatenate)(w740, w741) -> (w719:dbl[])
        n237 = Build Array (concatenate)(w739, w742) -> (w717:dbl[])
        n238 = local write "Is off"(w726) -> ()
        n239 = local write "Is on"(w725) -> ()
        n240 = Build Array (concatenate)(w781, w780) -> (w716:dbl[])
        n241 = Build Array (concatenate)(w768, w747) -> (w715:dbl[])
        n242 = Build Array (concatenate)(w744, w746) -> (w714:dbl[])
        n243 = Build Array (concatenate)(w743, w745) -> (w713:dbl[])
        n244 = Build Array (concatenate)(w732, w725) -> (w712:dbl[])
        n245 = Build Array (concatenate)(w731, w726) -> (w711:dbl[])
        n246 = Build Array (concatenate)(w754, w727) -> (w710:dbl[])
        n247 = Build Array (concatenate)(w755, w728) -> (w709:dbl[])
        n248 = Build Array (concatenate)(w736, w730) -> (w708:dbl[])
        n249 = Build Array (concatenate)(w735, w729) -> (w707:dbl[])
        n250 = local write "Ig off"(w729) -> ()
        n251 = local write "Ig on"(w730) -> ()
        n252 = local write "Id off"(w728) -> ()
        n253 = local write "Id on"(w727) -> ()
        n254 = call "4155C Split array.vi"("Number of VAR2 steps"=w718, "Y2 data in"=w710, "X data in"=w724, "Y1 data in"=w712, "Y3 data in"=w708, "error in (no error)"=w706) -> ("Array of clusters"=w722:cluster{"Y data in":dbl[], "X data in":dbl[]}[], "error out"=w705:errorcluster)  [unwired: 1 in]
        n255 = call "4155C Split array.vi"("Number of VAR2 steps"=w718, "Y2 data in"=w709, "X data in"=w724, "Y1 data in"=w711, "Y3 data in"=w707, "error in (no error)"=w705) -> ("Array of clusters"=w723:cluster{"Y data in":dbl[], "X data in":dbl[]}[], "error out"=w704:errorcluster)  [unwired: 1 in]
        n256 = call "4155C Split array.vi"("Number of VAR2 steps"=w718, "Y2 data in"=w716, "X data in"=w724, "Y1 data in"=w719, "Y3 data in"=w714, "error in (no error)"=w704) -> ("Array of clusters"=w772:cluster{"Y data in":dbl[], "X data in":dbl[]}[], "error out"=w703:errorcluster)  [unwired: 1 in]
        n257 = call "4155C Split array.vi"("Number of VAR2 steps"=w718, "Y2 data in"=w715, "X data in"=w724, "Y1 data in"=w717, "Y3 data in"=w713, "error in (no error)"=w703) -> ("Array of clusters"=w769:cluster{"Y data in":dbl[], "X data in":dbl[]}[], "error out"=w702:errorcluster)  [unwired: 1 in]
        n258 = Open/Create/Replace File(file path (use dialog)=w828, error in=w702, operation (0:open)=w783) -> (refnum out=w766:refnum<file>, error out=w764:errorcluster)  [unwired: 3 in, 1 out]
        n259 = call "4155C Make Big 2d array.vi"("1D Var1"=w782, "1d IS"=w749, "1d ID"=w751, "1d IG"=w748, "1d SMU4"=w786, "SMU4"=w785, "VAR2 START"=w787, "Number of VAR2 steps"=w718, "VAR2 STEP"=w788, "VAR1 Name"="Vd", "Decimal places in header"=i8 1, "VAR2 Name"="Vg") -> ("Header array"=w767:string[], "Data array"=w765:dbl[][])  [unwired: 14 in]
        n260 = local write "Imax vs time"(w772) -> ()
        n261 = local write "Imin vs time"(w769) -> ()
        n262 = local write "Ion vs time"(w722) -> ()
        n263 = local write "Ioff vs time"(w723) -> ()
        n264 = call "4155C Config Chart Colours.vi"("Numeric"=w718, "XY Graph 2"=w753) -> ()  [unwired: 6 in]
        n265 = call "4155C Config Chart Colours.vi"("Numeric"=w718, "XY Graph 2"=w752) -> ()  [unwired: 6 in]
        n266 = call "4155C Config Chart Colours.vi"("Numeric"=w718, "XY Graph 2"=w721) -> ()  [unwired: 6 in]
        n267 = call "4155C Config Chart Colours.vi"("Numeric"=w718, "XY Graph 2"=w720) -> ()  [unwired: 6 in]
        n268 = call "4155C Config Chart Colours.vi"("Numeric"=w718, "XY Graph 2"=w779) -> ()  [unwired: 6 in]
        n269 = call "4155C Write array to file.vi"("Byte Stream File Refnum"=w766, "Header"=w767, "Data Array"=w765, "error in (no error)"=w764) -> ("dup refnum"=w763:refnum<file>, "error out"=w762:errorcluster)  [unwired: 1 in]
        n270 = Close File(refnum=w763, error in=w762) -> (error out=w823:errorcluster)  [unwired: 1 out]
      }
      frame "output-fpp" {
        n271 = Number To Decimal String(number=w850) -> (decimal integer string=w904:string)  [unwired: 1 in]
        n272 = Bundle By Name(cluster=w880, "Emergency Stop"=w907) -> (w917:T2)
        n273 = Delete From Array(array=w895, index=0 ("Index")) -> (deleted portion=w893:string, array with subset deleted=w892:string[])  [unwired: 1 in]
        n274 = VISA Write(VISA resource name=w871, write buffer=":PAGE:CHAN:MODE SWE;" ("write buffer (\"\")"), error in (no error)=w868) -> (VISA resource name out=w870:refnum<visa-resource-name>, error out=w869:errorcluster)  [unwired: 1 out]
        n275 = Concatenate Strings(w903, "-outputfpp-" ("Substring"), w904, w849, ".txt" ("Substring")) -> (w906:string)
        n276 = case shown="\"d\", Default" w893 {
          tunnel: [w918 w919] -> w891
          frame "s" {
            w918 = u16 0 items=["Single", "Double"] ("sweep mode")
          }
          frame "d", Default {
            w919 = u16 1 items=["Single", "Double"] ("sweep mode")
          }
        }
        n277 = Fract/Exp String To Number(string=w892) -> (number=w874:dbl[])  [unwired: 3 in, 1 out]
        n278 = String To Path(string=w906) -> (path=w902:path)
        n279 = Index Array(array=w874, index #1=0 ("Index")) -> (element #1=w890:dbl, element #2=w889:dbl, element #3=w888:dbl)  [unwired: 2 in]
        n280 = Delete From Array(array=w874, length=3 ("Length"), index=0 ("Index")) -> (array with subset deleted=w873:dbl[])  [unwired: 1 out]
        n281 = Bundle By Name(cluster=w882, "Gate Start"=w890, "Gate Stop"=w889, "Gate Step (linear only)"=w888, "Gate Compliance"=w900, "Range mode"=w866, "Range"=w865) -> (w916:T6)
        n282 = Index Array(array=w873, index #1=0 ("Index")) -> (element #1=w885:dbl, element #2=w884:dbl, element #3=w883:dbl)  [unwired: 2 in]
        n283 = call <vilib>:"compatOverwrite.vi"("overwrite (F)"=TRUE) -> ("overwrite?"=w854:T8)
        n284 = Bundle By Name(cluster=w881, "Drain Start"=w885, "Drain Stop"=w884, "Drain Step"=w883, "Drain Compliance"=w901, "Range mode"=w864, "Range"=w867) -> (w915:T7)
        n285 = call "4155C Output-FPP.vi"("VISA resource name in"=w870, "Gate"=w916, "Drain"=w915, "Timings"=w899, "error in (no error)"=w869, "sweep mode"=w891, "Panel controls"=w917) -> ("VD"=w859:dbl[], "Outparams"=w862:T9, "VISA Resource Name out"=w897:refnum<visa-resource-name>, "Vprobe2"=w858:dbl[], "ID"=w857:dbl[], "IG"=w856:dbl[], "Vprobe1"=w855:dbl[], "error out"=w898:errorcluster)  [unwired: 13 in]
        n286 = Unbundle By Name(w862) -> ("V2 Step"=w863:dbl, "V2 Start"=w861:dbl, "Number of points"=w860:i32)
        n287 = Open/Create/Replace File(file path (use dialog)=w902, error in=w898, operation (0:open)=w854) -> (refnum out=w912:refnum<file>, error out=w913:errorcluster)  [unwired: 3 in, 1 out]
        n288 = call "4155C Make Big 2d array FPP.vi"("1D Var1"=w859, "1d ID"=w857, "1d Vp2"=w858, "1d IG"=w856, "1d Vp1"=w855, "VAR2 START"=w861, "Number of VAR2 steps"=w860, "VAR2 STEP"=w863, "VAR1 Name"="Vd", "Decimal places in header"=i8 1, "VAR2 Name"="Vg") -> ("Header array"=w908:string[], "Data array"=w909:dbl[][])  [unwired: 15 in]
        n289 = call "4155C Write array to file.vi"("Byte Stream File Refnum"=w912, "Header"=w908, "Data Array"=w909, "error in (no error)"=w913) -> ("dup refnum"=w910:refnum<file>, "error out"=w911:errorcluster)  [unwired: 1 in]
        n290 = Close File(refnum=w910, error in=w911) -> (error out=w896:errorcluster)  [unwired: 1 out]
      }
      frame "itime" {
        n291 = Delete From Array(array=w922, index=1) -> (deleted portion=w921:string)  [unwired: 1 in, 1 out]
        n292 = Delete From Array(array=w922, index=0 ("Index")) -> (deleted portion=w951:string)  [unwired: 1 in, 1 out]
        n293 = Fract/Exp String To Number(string=w921) -> (number=w920:dbl)  [unwired: 3 in, 1 out]
        n294 = case shown="\"l\"" w951 {
          tunnel: w950 -> [w956 w958 w962]
          tunnel: [w955 w957 w961] -> w943
          tunnel: w920 -> [w953 _ w960]
          frame "s" {
            w954 = u32 0 items=["short  ", "medium  ", "long  "] ("integration time 2")
            n295 = Bundle By Name(cluster=w956, "integration time"=w954, "Short/Long integration time"=w953) -> (w955:T5)
          }
          frame "m", Default {
            w959 = u32 1 items=["short  ", "medium  ", "long  "] ("integration time 2")
            n296 = Bundle By Name(cluster=w958, "integration time"=w959) -> (w957:T5)
          }
          frame "l" {
            w963 = u32 2 items=["short  ", "medium  ", "long  "] ("integration time 2")
            n297 = Bundle By Name(cluster=w962, "integration time"=w963, "Short/Long integration time"=w960) -> (w961:T5)
          }
        }
      }
      frame "pulsed" {
        n298 = Delete From Array(array=w992, index=0 ("Index")) -> (deleted portion=w993:string, array with subset deleted=w980:string[])  [unwired: 1 in]
        n299 = case shown="\"on\", Default" w993 {
          tunnel: w991 -> [w1003 w1006]
          tunnel: [w1002 w1005] -> w984
          tunnel: w980 -> [w1000 _]
          frame "on", Default {
            w1001 = u16 1 items=["Continuous", "Pulsed"] ("sweep method")
            n300 = Fract/Exp String To Number(string=w1000) -> (number=w998:dbl[])  [unwired: 3 in, 1 out]
            n301 = Index Array(array=w998, index #1=0 ("Index")) -> (element #1=w997:dbl, element #2=w996:dbl, element #3=w995:dbl)  [unwired: 2 in]
            n302 = Bundle By Name(cluster=w1003, "sweep method"=w1001, "Pulse period"=w997, "Base voltage"=w996, "Pulse width"=w995) -> (w1002:T5)
          }
          frame "off" {
            w1004 = u16 0 items=["Continuous", "Pulsed"] ("sweep method")
            n303 = Bundle By Name(cluster=w1006, "sweep method"=w1004) -> (w1005:T5)
          }
        }
      }
      frame "gaterangemode" {
        n304 = Delete From Array(array=w1033, index=0 ("Index")) -> (deleted portion=w1034:string)  [unwired: 1 in, 1 out]
        n305 = case shown="\"f\"" w1034 {
          tunnel: [w1036 w1037 w1038] -> w1023
          frame "a", Default {
            w1036 = u16 0 items=["Auto", "Limited", "Fixed"] ("Gate Range\nmode 2")
          }
          frame "f" {
            w1037 = u16 2 items=["Auto", "Limited", "Fixed"] ("Gate Range\nmode 2")
          }
          frame "l" {
            w1038 = u16 1 items=["Auto", "Limited", "Fixed"] ("Gate Range\nmode 2")
          }
        }
      }
      frame "gaterange" {
        (unwired) u8 11 items=["10fA  ", "100fA  ", "1nA  ", "10nA", "100nA", "1uA", "10uA", "100uA", "1mA", "10mA", "100mA", "1A"] ("Gate Range 2")
        n306 = Delete From Array(array=w1072, index=0 ("Index")) -> (deleted portion=w1062:string)  [unwired: 1 in, 1 out]
        n307 = Scan Value(string=w1062, format string="") -> (value=w1060:dbl)  [unwired: 1 in, 1 out]
        n308 = Logarithm Base 10(1:w1060) -> (0:w1059:dbl)
        n309 = Round To Nearest(number=w1059) -> (nearest integer value=w1058:dbl)
        n310 = Add(x=w1058, y=11.0) -> (x+y=w1056:dbl)
        n311 = To Unsigned Byte Integer(number=w1056) -> (unsigned 8bit integer=w1055:u8)
      }
      frame "drainrange" {
        (unwired) u8 11 items=["10fA  ", "100fA  ", "1nA  ", "10nA", "100nA", "1uA", "10uA", "100uA", "1mA", "10mA", "100mA", "1A"] ("Gate Range 2")
        n312 = Delete From Array(array=w1107, index=0 ("Index")) -> (deleted portion=w1098:string)  [unwired: 1 in, 1 out]
        n313 = Scan Value(string=w1098, format string="") -> (value=w1096:dbl)  [unwired: 1 in, 1 out]
        n314 = Logarithm Base 10(1:w1096) -> (0:w1095:dbl)
        n315 = Round To Nearest(number=w1095) -> (nearest integer value=w1094:dbl)
        n316 = Add(x=w1094, y=11.0) -> (x+y=w1092:dbl)
        n317 = To Unsigned Byte Integer(number=w1092) -> (unsigned 8bit integer=w1091:u8)
      }
      frame "drainrangemode" {
        n318 = Delete From Array(array=w1135, index=0 ("Index")) -> (deleted portion=w1136:string)  [unwired: 1 in, 1 out]
        n319 = case shown="\"f\"" w1136 {
          tunnel: [w1138 w1139 w1140] -> w1125
          frame "a", Default {
            w1138 = u16 0 items=["Auto", "Limited", "Fixed"] ("Gate Range\nmode 2")
          }
          frame "f" {
            w1139 = u16 2 items=["Auto", "Limited", "Fixed"] ("Gate Range\nmode 2")
          }
          frame "l" {
            w1140 = u16 1 items=["Auto", "Limited", "Fixed"] ("Gate Range\nmode 2")
          }
        }
      }
      frame "Error", Default {
      }
      frame "logfile" {
        n320 = Number To Decimal String(number=w1183) -> (decimal integer string=w1218:string)  [unwired: 1 in]
        n321 = Concatenate Strings(w1217, "logfile" ("Substring"), w1218, w1181, ".txt" ("Substring")) -> (w1215:string)
        n322 = String To Path(string=w1215) -> (path=w1188:path)
        n323 = Unbundle(w1214) -> ("integration time"=w1213:u32, "Short/Long integration time"=w1212:dbl, "hold time (sec)"=w1211:dbl, "delay time (sec)"=w1210:dbl, "Step Time (0 disables)"=w1209:dbl, "sweep method"=w1208:u16, "Pulse period"=w1207:dbl, "Base voltage"=w1206:dbl, "Pulse width"=w1205:dbl)
        n324 = Build Array(w1213, w1212, w1211, w1210, w1209, w1208, w1207, w1206, w1205, w1199, w1200, w1201, w1202, w1203, w1204) -> (w1192:dbl[])
        n325 = Insert Into Array(array=dbl[][] [] ("Input Array"), new element=w1192) -> (w1191:dbl[][])  [unwired: 2 in]
        n326 = call <vilib>:"compatOverwrite.vi"("overwrite (F)"=TRUE) -> ("overwrite?"=w1186:T8)
        n327 = Open/Create/Replace File(file path (use dialog)=w1188, error in=w1190, operation (0:open)=w1186) -> (refnum out=w1196:refnum<file>, error out=w1195:errorcluster)  [unwired: 3 in, 1 out]
        n328 = call "4155C Write array to file.vi"("Byte Stream File Refnum"=w1196, "Header"=string[] ["Int Time", "Short/Long Itime", "Hold time", "Delay time", "Step time", "Sweep method", "Pulse period", "Base Voltage", "Pulse width", "Drain compliance", "Gate compliance", "Gate range mode", "Gate range", "S/D range mode", "S/D range"], "Data Array"=w1191, "error in (no error)"=w1195) -> ("dup refnum"=w1198:refnum<file>, "error out"=w1197:errorcluster)  [unwired: 1 in]
        n329 = Close File(refnum=w1198, error in=w1197) -> (error out=w1189:errorcluster)  [unwired: 1 out]
      }
      frame "sample" {
        n330 = Number To Decimal String(number=w1236) -> (decimal integer string=w1284:string)  [unwired: 1 in]
        n331 = Fract/Exp String To Number(string=w1281) -> (number=w1242:dbl[])  [unwired: 3 in, 1 out]
        n332 = Concatenate Strings(w1259, "-sample-" ("Substring"), w1284, w1234, ".txt" ("Substring")) -> (w1282:string)
        n333 = Index Array(array=w1242, index=0 ("Index")) -> (element=w1279:dbl)
        n334 = String To Path(string=w1282) -> (path=w1263:path)
        n335 = Index Array(array=w1242, index=2 ("Index")) -> (element=w1275:dbl)
        n336 = Index Array(array=w1242, index=3 ("Index")) -> (element=w1244:dbl)
        n337 = Index Array(array=w1242, index=4 ("Index")) -> (element=w1241:dbl)
        n338 = call "4155C Config Sampling Measurements.vi"("Sampling interval"=w1241, "Sample time"=w1244, "Display on/off"=TRUE, "Timings"=w1250, "Num Points"=w1275, "error in (no error)"=w1286, "Drain Compliance"=w1285, "Gate Compliance"=w1260, "VISA session"=w1287) -> ("error out"=w1288:errorcluster, "dup VISA resource name"=w1289:refnum<visa-resource-name>)  [unwired: 1 in]
        n339 = Index Array(array=w1242, index=1 ("Index")) -> (element=w1276:dbl)
        n340 = call "4155C Take Sample.vi"("Emergency Stop"=w1256, "error in (no error)"=w1288, "Vd"=w1276, "Vg"=w1279, "VISA resource name in"=w1289) -> ("error out"=w1254:errorcluster, "Id"=w1291:dbl[], "Ig"=w1265:dbl[], "VISA Resource Name out"=w1252:refnum<visa-resource-name>, "Is"=w1290:dbl[], "Time"=w1269:dbl[])  [unwired: 1 in]
        n341 = Insert Into Array(array=dbl[][] [] ("Input Array"), new element=w1269) -> (w1268:dbl[][])  [unwired: 2 in]
        n342 = Insert Into Array(array=w1268, new element=w1265) -> (w1267:dbl[][])  [unwired: 2 in]
        n343 = Insert Into Array(array=w1267, new element=w1291) -> (w1266:dbl[][])  [unwired: 2 in]
        n344 = VISA Write(VISA resource name=w1252, write buffer=":DISP ON" ("write buffer (\"\")"), error in (no error)=w1254) -> (VISA resource name out=w1251:refnum<visa-resource-name>, error out=w1253:errorcluster)  [unwired: 1 out]
        n345 = Insert Into Array(array=w1266, new element=w1290) -> (w1258:dbl[][])  [unwired: 2 in]
        n346 = Transpose 2D Array(2D array=w1258) -> (transposed array=w1257:dbl[][])
        n347 = call <vilib>:"compatOverwrite.vi"("overwrite (F)"=TRUE) -> ("overwrite?"=w1239:T8)
        n348 = Open/Create/Replace File(file path (use dialog)=w1263, error in=w1253, operation (0:open)=w1239) -> (refnum out=w1272:refnum<file>, error out=w1271:errorcluster)  [unwired: 3 in, 1 out]
        n349 = call "4155C Write array to file.vi"("Byte Stream File Refnum"=w1272, "Header"=string[] ["Time /s", "Ig /A", "Id /A", "Is /A"], "Data Array"=w1257, "error in (no error)"=w1271) -> ("dup refnum"=w1274:refnum<file>, "error out"=w1273:errorcluster)  [unwired: 1 in]
        n350 = Close File(refnum=w1274, error in=w1273) -> (error out=w1261:errorcluster)  [unwired: 1 out]
      }
      frame "samplei" {
        n351 = Number To Decimal String(number=w1308) -> (decimal integer string=w1359:string)  [unwired: 1 in]
        n352 = Concatenate Strings(w1338, "-samplei-" ("Substring"), w1359, w1307, ".txt" ("Substring")) -> (w1357:string)
        n353 = Fract/Exp String To Number(string=w1356) -> (number=w1323:dbl[])  [unwired: 3 in, 1 out]
        n354 = String To Path(string=w1357) -> (path=w1341:path)
        n355 = Index Array(array=w1323, index=4 ("Index")) -> (element=w1317:dbl)
        n356 = Index Array(array=w1323, index=3 ("Index")) -> (element=w1318:dbl)
        n357 = Index Array(array=w1323, index=1 ("Index")) -> (element=w1320:dbl)
        n358 = Index Array(array=w1323, index=0 ("Index")) -> (element=w1321:dbl)
        n359 = Index Array(array=w1323, index=2 ("Index")) -> (element=w1319:dbl)
        n360 = call "4155C Config SamplingI Measurements.vi"("Sample time"=w1319, "Display on/off"=TRUE, "Timings"=w1330, "Num Points"=w1320, "error in (no error)"=w1361, "Sampling interval"=w1318, "VISA session"=w1362) -> ("error out"=w1363:errorcluster, "dup VISA resource name"=w1364:refnum<visa-resource-name>)  [unwired: 3 in]
        n361 = call "4155C Take SampleI.vi"("Emergency Stop"=w1335, "error in (no error)"=w1363, "Idg 2"=w1321, "Vdg compliance 2"=w1317, "VISA resource name in"=w1364) -> ("error out"=w1333:errorcluster, "Idg"=w1366:dbl[], "Vdg"=w1343:dbl[], "VISA Resource Name out"=w1331:refnum<visa-resource-name>, "Is"=w1365:dbl[], "Time"=w1347:dbl[])  [unwired: 1 in]
        n362 = Insert Into Array(array=dbl[][] [] ("Input Array"), new element=w1347) -> (w1346:dbl[][])  [unwired: 2 in]
        n363 = Insert Into Array(array=w1346, new element=w1343) -> (w1345:dbl[][])  [unwired: 2 in]
        n364 = Insert Into Array(array=w1345, new element=w1366) -> (w1344:dbl[][])  [unwired: 2 in]
        n365 = VISA Write(VISA resource name=w1331, write buffer=":DISP ON" ("write buffer (\"\")"), error in (no error)=w1333) -> (VISA resource name out=w1316:refnum<visa-resource-name>, error out=w1332:errorcluster)  [unwired: 1 out]
        n366 = Insert Into Array(array=w1344, new element=w1365) -> (w1337:dbl[][])  [unwired: 2 in]
        n367 = call <vilib>:"compatOverwrite.vi"("overwrite (F)"=TRUE) -> ("overwrite?"=w1311:T8)
        n368 = Open/Create/Replace File(file path (use dialog)=w1341, error in=w1332, operation (0:open)=w1311) -> (refnum out=w1350:refnum<file>, error out=w1349:errorcluster)  [unwired: 3 in, 1 out]
        n369 = Transpose 2D Array(2D array=w1337) -> (transposed array=w1336:dbl[][])
        n370 = call "4155C Write array to file.vi"("Byte Stream File Refnum"=w1350, "Header"=string[] ["Time /s", "Vdg /V", "Idg /A", "Is /A"], "Data Array"=w1336, "error in (no error)"=w1349) -> ("dup refnum"=w1352:refnum<file>, "error out"=w1351:errorcluster)  [unwired: 1 in]
        n371 = Close File(refnum=w1352, error in=w1351) -> (error out=w1314:errorcluster)  [unwired: 1 out]
        n372 = VISA Write(VISA resource name=w1316, write buffer=";:PAGE:SCON:STAN OFF;:PAGE:CHAN:VSU2:DIS;" ("write buffer (\"\")"), error in (no error)=w1314) -> (VISA resource name out=w1312:refnum<visa-resource-name>, error out=w1313:errorcluster)  [unwired: 1 out]
      }
      frame "#" {
        n373 = VISA Write(VISA resource name=w1387, write buffer=":DISP ON" ("write buffer (\"\")"), error in (no error)=w1386) -> (VISA resource name out=w1385:refnum<visa-resource-name>, error out=w1384:errorcluster)  [unwired: 1 out]
      }
      frame "stressV" {
        n374 = Number To Decimal String(number=w1411) -> (decimal integer string=w1452:string)  [unwired: 1 in]
        n375 = Concatenate Strings(w1436, "-stressV-" ("Substring"), w1452, w1410, ".txt" ("Substring")) -> (w1450:string)
        n376 = Fract/Exp String To Number(string=w1449) -> (number=w1422:dbl[])  [unwired: 3 in, 1 out]
        n377 = String To Path(string=w1450) -> (path=w1440:path)
        n378 = Index Array(array=w1422, index=3 ("Index")) -> (element=w1419:dbl)
        n379 = Index Array(array=w1422, index=1 ("Index")) -> (element=w1417:dbl)
        n380 = Index Array(array=w1422, index=0 ("Index")) -> (element=w1416:dbl)
        n381 = Index Array(array=w1422, index=4 ("Index")) -> (element=w1421:dbl)
        n382 = Index Array(array=w1422, index=2 ("Index")) -> (element=w1418:dbl)
        n383 = call "4155C Config V Stress.vi"("VISA session"=w1455, "ID compliance"=w1419, "VD"=w1417, "VG"=w1416, "IG compliance"=w1418, "error in (no error)"=w1454, "Display on/off"=TRUE) -> ("dup VISA resource name"=w1457:refnum<visa-resource-name>, "error out"=w1456:errorcluster)
        n384 = call "4155C Apply Stress.vi"("error in (no error)"=w1456, "Duration"=w1421, "Emergency Stop"=w1435, "VISA resource name in"=w1457) -> ("error out"=w1433:errorcluster, "VISA Resource Name out"=w1431:refnum<visa-resource-name>)
        n385 = VISA Write(VISA resource name=w1431, write buffer=":DISP ON" ("write buffer (\"\")"), error in (no error)=w1433) -> (VISA resource name out=w1430:refnum<visa-resource-name>, error out=w1432:errorcluster)  [unwired: 1 out]
        n386 = call <vilib>:"compatOverwrite.vi"("overwrite (F)"=TRUE) -> ("overwrite?"=w1415:T8)
        n387 = Open/Create/Replace File(file path (use dialog)=w1440, error in=w1432, operation (0:open)=w1415) -> (refnum out=w1443:refnum<file>, error out=w1442:errorcluster)  [unwired: 3 in, 1 out]
        n388 = call "4155C Write array to file.vi"("Byte Stream File Refnum"=w1443, "Header"=string[] ["V stress completed successfully", ""], "error in (no error)"=w1442) -> ("dup refnum"=w1445:refnum<file>, "error out"=w1444:errorcluster)  [unwired: 2 in]
        n389 = Close File(refnum=w1445, error in=w1444) -> (error out=w1438:errorcluster)  [unwired: 1 out]
      }
      frame "stressI" {
        n390 = Number To Decimal String(number=w1473) -> (decimal integer string=w1510:string)  [unwired: 1 in]
        n391 = Concatenate Strings(w1494, "-stressI-" ("Substring"), w1510, w1472, ".txt" ("Substring")) -> (w1508:string)
        n392 = Fract/Exp String To Number(string=w1507) -> (number=w1482:dbl[])  [unwired: 3 in, 1 out]
        n393 = Index Array(array=w1482, index=1 ("Index")) -> (element=w1478:dbl)
        n394 = Index Array(array=w1482, index=0 ("Index")) -> (element=w1479:dbl)
        n395 = call "4155C Config I Stress.vi"("VISA session"=w1513, "IDG"=w1479, "VDG compliance"=w1478, "error in (no error)"=w1512, "Display on/off"=TRUE) -> ("dup VISA resource name"=w1515:refnum<visa-resource-name>, "error out"=w1514:errorcluster)
        n396 = Index Array(array=w1482, index=2 ("Index")) -> (element=w1480:dbl)
        n397 = String To Path(string=w1508) -> (path=w1498:path)
        n398 = call "4155C Apply Stress.vi"("error in (no error)"=w1514, "Duration"=w1480, "Emergency Stop"=w1493, "VISA resource name in"=w1515) -> ("error out"=w1491:errorcluster, "VISA Resource Name out"=w1489:refnum<visa-resource-name>)
        n399 = VISA Write(VISA resource name=w1489, write buffer=":DISP ON" ("write buffer (\"\")"), error in (no error)=w1491) -> (VISA resource name out=w1488:refnum<visa-resource-name>, error out=w1490:errorcluster)  [unwired: 1 out]
        n400 = call <vilib>:"compatOverwrite.vi"("overwrite (F)"=TRUE) -> ("overwrite?"=w1477:T8)
        n401 = Open/Create/Replace File(file path (use dialog)=w1498, error in=w1490, operation (0:open)=w1477) -> (refnum out=w1501:refnum<file>, error out=w1500:errorcluster)  [unwired: 3 in, 1 out]
        n402 = call "4155C Write array to file.vi"("Byte Stream File Refnum"=w1501, "Header"=string[] ["I stress completed successfully", ""], "error in (no error)"=w1500) -> ("dup refnum"=w1503:refnum<file>, "error out"=w1502:errorcluster)  [unwired: 2 in]
        n403 = Close File(refnum=w1503, error in=w1502) -> (error out=w1496:errorcluster)  [unwired: 1 out]
      }
      frame "vsu2pulse" {
        n404 = Number To Decimal String(number=w1531) -> (decimal integer string=w1566:string)  [unwired: 1 in]
        n405 = Concatenate Strings(w1551, "-vsu2-" ("Substring"), w1566, w1530, ".txt" ("Substring")) -> (w1564:string)
        n406 = Fract/Exp String To Number(string=w1563) -> (number=w1539:dbl[])  [unwired: 3 in, 1 out]
        n407 = String To Path(string=w1564) -> (path=w1555:path)
        n408 = Index Array(array=w1539, index=1 ("Index")) -> (element=w1538:dbl)
        n409 = Index Array(array=w1539, index=0 ("Index")) -> (element=w1536:dbl)
        n410 = call "4155C Config VSU2 Stress.vi"("error in (no error)"=w1568, "VSU2"=w1536, "Display on/off"=TRUE, "VISA session"=w1569) -> ("error out"=w1570:errorcluster, "dup VISA resource name"=w1571:refnum<visa-resource-name>)
        n411 = call "4155C Apply Stress.vi"("error in (no error)"=w1570, "Duration"=w1538, "Emergency Stop"=w1550, "VISA resource name in"=w1571) -> ("error out"=w1548:errorcluster, "VISA Resource Name out"=w1546:refnum<visa-resource-name>)
        n412 = VISA Write(VISA resource name=w1546, write buffer=":DISP ON" ("write buffer (\"\")"), error in (no error)=w1548) -> (VISA resource name out=w1545:refnum<visa-resource-name>, error out=w1547:errorcluster)  [unwired: 1 out]
        n413 = call <vilib>:"compatOverwrite.vi"("overwrite (F)"=TRUE) -> ("overwrite?"=w1535:T8)
        n414 = Open/Create/Replace File(file path (use dialog)=w1555, error in=w1547, operation (0:open)=w1535) -> (refnum out=w1558:refnum<file>, error out=w1557:errorcluster)  [unwired: 3 in, 1 out]
        n415 = call "4155C Write array to file.vi"("Byte Stream File Refnum"=w1558, "Header"=string[] ["VSU2 pulse completed successfully", ""], "error in (no error)"=w1557) -> ("dup refnum"=w1560:refnum<file>, "error out"=w1559:errorcluster)  [unwired: 2 in]
        n416 = Close File(refnum=w1560, error in=w1559) -> (error out=w1553:errorcluster)  [unwired: 1 out]
      }
      frame "sample-fpp" {
        w1598 = string[] ["Time /s", "Id VgVd /A", "Ig VgVd /A", "Vp1 VgVd /V", "Vp2 VgVd /V"] ("Header")
        w1602 = "%d" ("format string")
        n417 = Number To Decimal String(number=w1587) -> (decimal integer string=w1650:string)  [unwired: 1 in]
        n418 = Fract/Exp String To Number(string=w1647) -> (number=w1635:dbl[])  [unwired: 3 in, 1 out]
        n419 = Concatenate Strings(w1641, "-samplefpp-" ("Substring"), w1650, w1586, ".txt" ("Substring")) -> (w1648:string)
        n420 = String To Path(string=w1648) -> (path=w1610:path)
        n421 = Index Array(array=w1635, index=0 ("Index")) -> (element=w1596:dbl)
        n422 = Index Array(array=w1635, index=1 ("Index")) -> (element=w1595:dbl)
        n423 = Index Array(array=w1635, index=2 ("Index")) -> (element=w1643:dbl)
        n424 = Index Array(array=w1635, index=3 ("Index")) -> (element=w1633:dbl)
        n425 = call "4155C Config Sampling Measurements FPP.vi"("VISA session"=w1653, "Num Points"=w1643, "Vg"=w1596, "Display on/off"=TRUE, "Gate Compliance"=w1642, "Drain Compliance"=w1651, "Standby"="Standby", "error in (no error)"=w1652, "Timings"=w1640, "Vd"=w1595, "Sample time"=w1633) -> ("dup VISA resource name"=w1612:refnum<visa-resource-name>, "error out"=w1611:errorcluster)  [unwired: 3 in]
        n426 = Number To Decimal String(number=w1596) -> (decimal integer string=w1622:string)  [unwired: 1 in]
        n427 = call "4155C Take Sample FPP.vi"("VISA resource name in"=w1612, "error in (no error)"=w1611, "Emergency Stop"=w1613) -> ("Time"=w1617:dbl[], "Vp1"=w1627:dbl[], "VISA Resource Name out"=w1593:refnum<visa-resource-name>, "Ig"=w1615:dbl[], "Id"=w1616:dbl[], "Vp2"=w1625:dbl[], "error out"=w1614:errorcluster)  [unwired: 10 in]
        n428 = Insert Into Array(array=dbl[][] [] ("Input Array"), new element=w1617) -> (w1631:dbl[][])  [unwired: 2 in]
        n429 = Number To Decimal String(number=w1595) -> (decimal integer string=w1620:string)  [unwired: 1 in]
        n430 = Insert Into Array(array=w1631, new element=w1616) -> (w1630:dbl[][])  [unwired: 2 in]
        n431 = Concatenate Strings("(Vg = " ("Substring"), w1622, "V, Vd = " ("Substring"), w1620, "V)" ("Substring")) -> (w1618:string)
        n432 = Insert Into Array(array=w1630, new element=w1615) -> (w1629:dbl[][])  [unwired: 2 in]
        n433 = Insert Into Array(array=w1629, new element=w1627) -> (w1626:dbl[][])  [unwired: 2 in]
        n434 = Insert Into Array(array=w1626, new element=w1625) -> (w1594:dbl[][])  [unwired: 2 in]
        n435 = Transpose 2D Array(2D array=w1594) -> (transposed array=w1624:dbl[][])
        n436 = call <vilib>:"compatOverwrite.vi"("overwrite (F)"=TRUE) -> ("overwrite?"=w1591:T8)
        n437 = Open/Create/Replace File(file path (use dialog)=w1610, error in=w1614, operation (0:open)=w1591) -> (refnum out=w1607:refnum<file>, error out=w1608:errorcluster)  [unwired: 3 in, 1 out]
        n438 = Array To Spreadsheet String(array=w1598, 3:w1602) -> (spreadsheet string=w1604:string)  [unwired: 1 in]
        n439 = Search and Replace String(replace all?=TRUE ("replace all? (F)"), input string=w1604, search string="VgVd", replace string=w1618) -> (result string=w1600:string)  [unwired: 4 in, 3 out]
        n440 = Spreadsheet String To Array(format string=w1602, spreadsheet string=w1600, array type (2D Dbl)=w1598) -> (array=w1599:string[])  [unwired: 1 in]
        n441 = call "4155C Write array to file.vi"("Byte Stream File Refnum"=w1607, "Header"=w1599, "Data Array"=w1624, "error in (no error)"=w1608) -> ("dup refnum"=w1605:refnum<file>, "error out"=w1606:errorcluster)  [unwired: 1 in]
        n442 = Close File(refnum=w1605, error in=w1606) -> (error out=w1592:errorcluster)  [unwired: 1 out]
      }
      frame "resample-fpp" {
        w1682 = string[] ["Time /s", "Id VgVd /A", "Ig VgVd /A", "Vp1 VgVd /V", "Vp2 VgVd /V"] ("Header")
        w1686 = "%d" ("format string")
        n443 = Number To Decimal String(number=w1668) -> (decimal integer string=w1726:string)  [unwired: 1 in]
        n444 = Fract/Exp String To Number(string=w1723) -> (number=w1675:dbl[])  [unwired: 3 in, 1 out]
        n445 = Concatenate Strings(w1719, "-resamplefpp-" ("Substring"), w1726, w1669, ".txt" ("Substring")) -> (w1724:string)
        n446 = String To Path(string=w1724) -> (path=w1694:path)
        n447 = Index Array(array=w1675, index=0 ("Index")) -> (element=w1681:dbl)
        n448 = Index Array(array=w1675, index=1 ("Index")) -> (element=w1680:dbl)
        n449 = Number To Decimal String(number=w1681) -> (decimal integer string=w1704:string)  [unwired: 1 in]
        n450 = call "4155C Take Sample FPP.vi"("VISA resource name in"=w1677, "error in (no error)"=w1676, "Emergency Stop"=w1695) -> ("Time"=w1699:dbl[], "Vp1"=w1709:dbl[], "VISA Resource Name out"=w1679:refnum<visa-resource-name>, "Ig"=w1697:dbl[], "Id"=w1698:dbl[], "Vp2"=w1707:dbl[], "error out"=w1696:errorcluster)  [unwired: 10 in]
        n451 = Insert Into Array(array=dbl[][] [] ("Input Array"), new element=w1699) -> (w1713:dbl[][])  [unwired: 2 in]
        n452 = Number To Decimal String(number=w1680) -> (decimal integer string=w1702:string)  [unwired: 1 in]
        n453 = Insert Into Array(array=w1713, new element=w1698) -> (w1712:dbl[][])  [unwired: 2 in]
        n454 = Concatenate Strings("(Vg = " ("Substring"), w1704, "V, Vd = " ("Substring"), w1702, "V)" ("Substring")) -> (w1700:string)
        n455 = Insert Into Array(array=w1712, new element=w1697) -> (w1711:dbl[][])  [unwired: 2 in]
        n456 = Insert Into Array(array=w1711, new element=w1709) -> (w1708:dbl[][])  [unwired: 2 in]
        n457 = Insert Into Array(array=w1708, new element=w1707) -> (w1674:dbl[][])  [unwired: 2 in]
        n458 = call <vilib>:"compatOverwrite.vi"("overwrite (F)"=TRUE) -> ("overwrite?"=w1673:T8)
        n459 = Open/Create/Replace File(file path (use dialog)=w1694, error in=w1696, operation (0:open)=w1673) -> (refnum out=w1691:refnum<file>, error out=w1692:errorcluster)  [unwired: 3 in, 1 out]
        n460 = Array To Spreadsheet String(array=w1682, 3:w1686) -> (spreadsheet string=w1688:string)  [unwired: 1 in]
        n461 = Transpose 2D Array(2D array=w1674) -> (transposed array=w1706:dbl[][])
        n462 = Search and Replace String(replace all?=TRUE ("replace all? (F)"), input string=w1688, search string="VgVd", replace string=w1700) -> (result string=w1684:string)  [unwired: 4 in, 3 out]
        n463 = Spreadsheet String To Array(format string=w1686, spreadsheet string=w1684, array type (2D Dbl)=w1682) -> (array=w1683:string[])  [unwired: 1 in]
        n464 = call "4155C Write array to file.vi"("Byte Stream File Refnum"=w1691, "Header"=w1683, "Data Array"=w1706, "error in (no error)"=w1692) -> ("dup refnum"=w1689:refnum<file>, "error out"=w1690:errorcluster)  [unwired: 1 in]
        n465 = Close File(refnum=w1689, error in=w1690) -> (error out=w1678:errorcluster)  [unwired: 1 out]
      }
      frame "serial" {
        n466 = local read "Termination char\n(0xA = '\\n' = LF)\n(0xD = '\\r' = CR)"() -> (w1749:u8)
        n467 = local read "Enable Termination\nChar (T)"() -> (w1750:bool)
        n468 = Index Array(array=w1757, index=0 ("Index")) -> (element=w1756:string)
        n469 = local read "parity"() -> (w1740:u16)
        n470 = local read "Delay before read (ms)"() -> (w1751:u32)
        n471 = local read "byte count"() -> (w1748:u32)
        n472 = local read "Timeout (ms)"() -> (w1747:u32)
        n473 = local read "VISA resource name"() -> (w1744:refnum<visa-resource-name>)
        n474 = local read "baud rate"() -> (w1743:u32)
        n475 = local read "Serial End Mode for Reads"() -> (w1742:u16)
        n476 = local read "data bits"() -> (w1741:u16)
        n477 = local read "stop bits"() -> (w1746:u16)
        n478 = local read "flow control"() -> (w1745:u16)
        n479 = call "Serial write and read v0.5.vi"("Delay before read (ms)"=w1751, "Termination char\n(0xA = '\\n' = LF)\n(0xD = '\\r' = CR)"=w1749, "Enable Termination\nChar (T)"=w1750, "parity"=w1740, "stop bits"=w1746, "string to write"=w1756, "flow control"=w1745, "byte count"=w1748, "Serial Settings:Serial End Mode for Reads"=w1742, "Timeout (ms)"=w1747, "error in (no error)"=w1762, "VISA resource name"=w1744, "baud rate"=w1743, "data bits"=w1741) -> ("Serial port output"=w1752:string, "error out"=w1761:errorcluster)
        n480 = Build Array (concatenate)(w1752, w1753) -> (w1754:string[])
      }
    }
    n481 = local read "Time Units"() -> (w61:u16)
    n482 = case shown="0" w61 {
      tunnel: ["Time (Seconds)" ("element") "Time (Minutes)" ("element") "Time (Hours)" ("element")] -> w101
      frame 0 {
      }
      frame 1, Default {
      }
      frame 2 {
      }
    }
    n483 = Build Array(w114, w69, w79, w78, w77, w76, w75, w74, w73, w72, w71, w70, w68) -> (w138:dbl[][])
    n484 = Transpose 2D Array(2D array=w138) -> (transposed array=w137:dbl[][])
    n485 = Concatenate Strings(w66, "-Imax_Imin_Ion_Ioff_vs_time.txt" ("Suffix (Imax,Imin,Ion,Ioff)")) -> (w148:string)
    n486 = Build Array(w101, "Is max (A)" ("VAR2 Name"), "Is min (A)" ("VAR2 Name"), "Id max (A)" ("VAR2 Name"), "Id min (A)" ("VAR2 Name"), "Ig max (A)" ("VAR2 Name"), "Ig min (A)" ("VAR2 Name"), "Is on (A)" ("VAR2 Name"), "Is off (A)" ("VAR2 Name"), "Id on (A)" ("VAR2 Name"), "Id off (A)" ("VAR2 Name"), "Ig on (A)" ("VAR2 Name"), "Ig off (A)" ("VAR2 Name")) -> (w143:string[])
    n487 = Array To Spreadsheet String(array=w137, 3:"%e" ("format string")) -> (spreadsheet string=w141:string)  [unwired: 1 in]
    n488 = Array To Spreadsheet String(array=w143, 3:"" ("format string")) -> (spreadsheet string=w142:string)  [unwired: 1 in]
    n489 = String To Path(string=w148) -> (path=w147:path)
    n490 = Build Array(w142, w141) -> (w140:string[])
    n491 = Write to Text File(file (use dialog)=w147, text=w140, error in=w112) -> (refnum out=w149:refnum<file>, error out=w139:errorcluster)  [unwired: 1 in, 1 out]
    n492 = Close File(refnum=w149, error in=w139) -> (error out=w65:errorcluster)  [unwired: 1 out]
    n493 = Concatenate Strings(w66, "-serial_port_output.txt" ("Suffix (serial port log)")) -> (w118:string)
    n494 = String To Path(string=w118) -> (path=w117:path)
    n495 = Build Array(w101, "Serial port input" ("VAR2 Name"), "Serial port output: ") -> (w105:string[])
    n496 = Array To Spreadsheet String(array=w109, 3:"" ("format string")) -> (spreadsheet string=w102:string)  [unwired: 1 in]
    n497 = Array To Spreadsheet String(array=w105, 3:"" ("format string")) -> (spreadsheet string=w103:string)  [unwired: 1 in]
    n498 = Build Array(w103, w102) -> (w104:string[])
    n499 = Array To Spreadsheet String(array=w108, 3:"" ("format string")) -> (spreadsheet string=w123:string)  [unwired: 1 in]
    n500 = Write to Text File(file (use dialog)=w117, text=w104, error in=w65) -> (refnum out=w119:refnum<file>, error out=w120:errorcluster)  [unwired: 1 in, 1 out]
    n501 = Close File(refnum=w119, error in=w120) -> (error out=w63:errorcluster)  [unwired: 1 out]
    n502 = local write "Serial port data"(w123) -> ()
  }
  "error out" <- w24
  "Timings Indicator" <- w12
  "Is max" <- w6
  "Id max" <- w6
  "Ig max" <- w6
  "Imax vs time" <- w2
  "I vs Vg" <- w2
  "Imin vs time" <- w2
  "I vs Vd" <- w2
  "Serial port data" <- "" ("Serial port data")
  "Is min" <- w5
  "Id min" <- w5
  "Ig min" <- w5
  "Ion vs time" <- w2
  "Ioff vs time" <- w2
  "Is on" <- w4
  "Id on" <- w4
  "Ig on" <- w4
  "Is off" <- w3
  "Id off" <- w3
  "Ig off" <- w3
